vi "PECT - Scan_time gate.vi"() -> ()   [LabVIEW 2012]
uses:
  <vilib>/DAQmx/write.llb/DAQmx Write (Analog 1D Wfm NChan NSamp).vi
  <vilib>/DAQmx/read.llb/DAQmx Read (Analog 1D DBL 1Chan NSamp).vi
  <vilib>/DAQmx/read.llb/DAQmx Read (Analog Wfm 1Chan NSamp).vi
  <vilib>/Instr/_visa.llb/VISA Configure Serial Port (Instr).vi
  <vilib>/DAQmx/create/channels.llb/DAQmx Create Channel (AI-Voltage-Basic).vi
  <vilib>/DAQmx/configure/timing.llb/DAQmx Timing (Sample Clock).vi
  <vilib>/DAQmx/configure/task.llb/DAQmx Configure Logging (TDMS).vi
  <vilib>/DAQmx/configure/trigger.llb/DAQmx Start Trigger (Digital Edge).vi
  <vilib>/DAQmx/create/channels.llb/DAQmx Create Channel (AO-Voltage-Basic).vi
  <vilib>/DAQmx/miscellaneous.llb/DAQmx Fill In Error Info.vi
  Global_data.vi
  <vilib>/express/express analysis/Spectral/Block/exnSpectralBlock spectral measurements PSD poly.vi
  <vilib>/express/express analysis/Spectral/Block/exnSpectralBlock spectral measurements PSD WFM.vi
  <vilib>/express/express analysis/Spectral/XNode/ExpressSpectralMeasurementsBlockNode.xnode
  <resource>/objmgr/daqmx.rc
  <vilib>/measure/NI_MABase.lvlib
  <vilib>/Platform/NI_3dgraph.lvlib
panel:
  in  "Gate 2":dbl=2.0
  in  "Gate 1":dbl=4.0
  in  "Backward scan":bool
  in  "X-length count":dbl=20.0
  out "No.data":i32
  in  "Save Scan mode":bool caption="Save Process"
  in  "Plot style":i32(ring)=5 items=["cwLine"=1, "cwPoint"=2, "cwLinePoint"=3, "cwHiddenLine"=4, "cwSurface"=5, "cwSurfaceLine"=6, "cwSurfaceNormal"=7, "cwContourLine"=8, "cwSurfaceContour"=9]
  in  "Stop 4":bool
  in  "Forward scan":bool
  in  "ViewMode":i32(ring) items=["cwViewXYPlane", "cwViewXZPlane", "cwViewYZPlane", "cwViewUserDefined"]
  in  "Stop Scan 2":bool
  in  "Emergency Stop":bool
  in  "Stop 3":bool
  in  "Home Y":bool
  in  "Home X":bool
  in  "Back":bool
  in  "Front":bool
  in  "Left":bool
  in  "Right":bool
  in  "Stop Scan":bool
  in  "Move Distance (mm)":dbl=10.0
  in  "Scan":bool
  in  "Pulser Trigger Source":tag="/Dev1/PFI1" caption="소스"
  in  "Open":bool
  in  "Tab Control 2":T1(tab)
  out "Hall sensors signal":waveform(dbl)[](graph)=[{"t0"=timestamp(3525645621.636764 s since 1904-01-01), "dt"=1.9999999999999944e-06, "Y"=array[2100 elements], "attributes"=variant("NI_ChannelName"=variant(string "Dev1/ai0"), "NI_UnitDescription"=variant(string "Volts"))}, {"t0"=timestamp(3525645621.636764 s since 1904-01-01), "dt"=1.9999999999999944e-06, "Y"=array[2100 elements], "attributes"=variant("NI_ChannelName"=variant(string "Dev1/ai0"), "NI_UnitDescription"=variant(string "Volts"))}]
  out "Feature Extraction":dbl(graph)=0.021153968958947764
  out "Waveform Graph 2":waveform(dbl)[](graph)=[{"t0"=timestamp(0 s since 1904-01-01), "dt"=1.25e-06, "Y"=array[8000 elements]}]
  out "Power spectral density":cluster{"f0":dbl, "df":dbl, "magnitude":dbl[]}[](graph)=[{"f0"=0.0, "df"=238.09523809523876, "magnitude"=[-25.4340272409559, -28.495970805276507, -69.09064054555873, -79.11355871279994, -75.69366097931027, -84.18131507822396, -80.50168881348966, -82.72314293089615, -87.19630499623688, -82.83568021481967, -89.95290866002237, -85.90392585035596, -87.41269111550386, -91.40893948681482, -86.69370819914215, -93.36336146616782, -89.019380476413, -89.73232030153878, -94.58261196624535, -89.16287927388944, -94.965890302584, -91.86846413178648, -91.95327957161693, -97.62687167891286, -91.59993648735762, -97.30685711015555, -93.8350762480425, -93.27921214218685, -99.59438563802183, -93.1824258709588, -98.3113125531512, -95.45425138584356, -94.39327135467576, -100.65352961491782, -94.55889081970952, -99.40788907105079, -97.93617495318924, -96.19517579047603, -103.97036797797732, -96.40295202889732, -99.7036956909043, -99.48760137175819, -97.46192979187015, -106.29271483151813, -97.51447379981207, -99.86179280251669, -100.43811038443037, -97.59011642740829, -105.58363666166275, -99.01126121197593, -101.01575323613292, -101.90167607549864, -98.61952569586691, -106.73670466995647, -99.29976101634999, -101.54959604687718, -105.17330050767885, -100.09392305285375, -109.78264848704497, -100.98914236173123, -101.81665207962125, -105.42358374403365, -99.82880728595141, -107.07330885402075, -101.07712607444097, -101.03780825357597, -107.32811151840846, -101.221643458408, -105.63776326231454, -101.8420593566944, -101.80081629073969, -107.47915505307212, -101.12986632760553, -106.84901404755908, -102.73715610491038, -101.51552854007832, -107.28771371003282, -101.3928633472346, -107.44515355816633, -104.89304864643535, -103.1455098860718, -110.19910428997925, -102.73063833081197, -107.57101838377707, -104.90574568581201, -103.72599931018533, -109.97178587260123, -103.24611921258705, -108.36098023558972, -106.6408311450923, -104.73569536588386, -116.21683530762306, -105.02627439976544, -107.15856030450797, -109.81191038702062, -105.53476822084077, -119.10077766590356, -105.31867536160968, -106.9718410299748, -108.34458911268797, -104.70307996109247, -114.76704583683203, -106.29948298493936, -108.55077108437321, -112.16618350190343, -105.98453547558171, -114.68576835450673, -107.50968901677987, -107.89174277914348, -111.59875709602721, -106.69368240333122, -114.93273233954758, -105.23904516482949, -106.00272331017348, -110.36103151258544, -104.93177986717492, -110.8835476773746, -106.69346348818806, -106.66103973993782, -119.11729839814336, -108.06338160849775, -114.5879267769655, -108.59816838472844, -107.53189260743514, -114.07390818184973, -106.70996756049796, -113.27381274118753, -109.50270539577696, -107.37282420343303, -113.4779718725949, -106.04267666963091, -111.30294425571472, -112.46717993668915, -109.13164915488709, -116.65287200885172, -107.03002573045511, -110.21479040603631, -112.476075561056, -106.97710947409149, -119.42145279296255, -108.3200486628316, -110.46641858585929, -117.16650627564961, -109.73297826697552, -120.31689830731365, -107.19513745371916, -110.66663569403087, -113.30365980039964, -110.01971553524372, -123.68660617105166, -110.8171755739396, -111.11382172813546, -117.76239209582961, -109.49899370205401, -115.22252846498625, -111.1932077339224, -112.38235939086871, -118.22207022901702, -110.6546796895719, -116.97450780644367, -110.82401674194465, -111.96705198878843, -118.28092956599232, -110.5621503678909, -121.25720613496851, -111.98371482341479, -113.27928013246557, -111.96833712758355, -108.56859286664552, -120.32790468431601, -110.82699792221703, -110.79062667340345, -122.65756767769517, -110.48843456045427, -116.8782055296399, -115.43719816168479, -114.47619780315773, -121.42183196132746, -111.60631415727042, -120.68077308056417, -109.35478690141552, -109.03210709352732, -120.6260555904793, -109.47936424950136, -113.33719701518146, -112.88325992990137, -110.99901978536154, -123.19636626521421, -109.09861317900774, -113.33125158106256, -115.35673297389727, -112.77249677632989, -124.61163141716472, -114.68140920359865, -121.89642913325117, -115.47413298424323, -112.82196063671608, -127.87542521315149, -111.54178118788309, -113.6448752704395, -120.76569423868874, -112.98651214877823, -123.18868565400437, -115.41399838634062, -115.46853076016815, -116.40989072804102, -110.69611347288615, -132.23164080331392, -114.76376391429793, -121.7246597336247, -117.46893009589195, -114.01899156779395, -125.22079066032327, -114.59524199183258, -114.50034890537415, -122.9532092227648, -113.72727798159212, -125.65163915514907, -113.4793801211504, -110.4090756414644, -125.63592649005872, -114.22938378193007, -116.74947251106808, -121.60535557984142, -116.79385283402802, -122.44667696630361, -113.43873413563811, -123.28159708694415, -113.92892974938164, -114.01193823589753, -121.62751955742443, -118.76839573694522, -125.52998605097204, -115.19609643487229, -117.49409595176479, -117.08423885198002, -119.48314867245172, -125.01675515413412, -117.92668164142911, -115.55962389856793, -125.63488616674975, -119.11862859365166, -114.78860770332909, -117.18339781294443, -111.18063004722558, -118.31775966044624, -111.6867367949252, -114.57226159377, -119.36541212960576, -113.90245139442648, -132.46343443313128, -120.1282759002165, -121.05279009698619, -118.9115822659523, -121.23280439248342, -116.31914159559688, -127.38829313950257, -117.34673005740623, -115.95249861902771, -114.9301657394146, -123.22361802797445, -110.83274939062106, -116.16624248562111, -116.76753364192771, -113.94454545069023, -122.95736945775944, -118.66755800656253, -129.1462641201204, -116.6351050110328, -117.22529407303742, -123.80212197360244, -115.89792176423389, -114.25823938606595, -125.60467961977515, -114.59958849364433, -121.70071005514421, -118.25968972451209, -114.69929400946009, -123.88209034116528, -115.03869272537257, -117.52034211782204, -115.27990843516797, -117.85366603932033, -125.16865559622727, -118.21960424638507, -119.69008755413566, -117.24640963460672, -114.32867295013791, -119.1576982419508, -122.85495988425586, -116.3373010103401, -114.53730203699834, -115.67017599990201, -127.144321037601, -115.73849102686786, -117.7626163106355, -119.7346592991025, -117.41317517684553, -125.0417974461613, -114.5488949833583, -116.59812516173781, -119.91064563147799, -115.27933218667663, -122.09990513751134, -120.95678574143693, -123.25641714743752, -112.5173710452192, -113.53735878806998, -129.23914933506734, -116.27157269711533, -148.4020512032711, -118.84888216023774, -123.82550527215588, -116.87770979616658, -111.32191810025745, -124.32675905891588, -114.37182733794062, -121.10713785851372, -122.59698730059695, -116.38346694563282, -121.69144349152856, -119.00883142493832, -110.81886738196273, -120.7909830607913, -115.01780448665316, -114.52055121633796, -132.6824191654361, -116.330695115645, -126.4664151018508, -118.32717907779282, -118.7288071595281, -120.42749846140066, -112.53185615773879, -124.26026008984286, -114.24089252048742, -120.00368190003405, -114.71738500842926, -112.92262025927133, -129.21127897188563, -113.5947811765517, -117.80802009651353, -117.0133790103226, -112.19210322760304, -118.17549968071762, -119.3256187825503, -118.84981507334446, -121.39118969751144, -114.64543555194373, -119.84814933224528, -114.09123407848944, -116.22899352170892, -116.41650104077173, -113.70057202673476, -124.52773908304957, -114.87372641784933, -116.11651108221098, -121.68680962246994, -115.78306007961302, -122.22621008657796, -118.81157995182392, -113.9402115821658, -132.636729517989, -114.49554876936634, -119.50980190398928, -123.27410972236837, -118.52851881066383, -122.25212982572599, -117.13947036230024, -120.85005588797962, -118.41526503460501, -117.61788553858068, -126.3872056783977, -114.98198608543298, -119.7789938911847, -120.84873579392627, -114.38831474301695, -153.35954756825245, -113.19505610638078, -114.17454820985151, -127.41069917723112, -114.92677241657191, -125.49053973810628, -113.36382196587914, -119.96785250843519, -122.47388530423243, -116.38671253508838, -120.0905790211523, -119.83326265062107, -117.88168146696918, -122.3132169880757, -115.87324909105399, -125.92003267803432, -113.96860176867415, -114.49156118371398, -127.52634390035722, -115.05967156528004, -126.82020221981517, -117.93643187259194, -116.51163213641807, -119.47551219110167, -119.55225172256931, -116.9512257852571, -122.23153124485954, -120.8368476753637, -121.48473913072222, -115.83122660909913, -135.74260014140523, -116.58358375805423, -118.15236945484727, -119.06674062398864, -115.7844834762477, -125.06111738611818, -114.7801535050972, -115.2696605691888, -123.98656374010793, -119.29025555731172, -118.29146803784099, -119.55696172158135, -118.06884171238352, -127.81587648134607, -120.41730580797976, -123.49626136731604, -112.2147141798107, -116.22555232584983, -132.79419178871254, -119.66964883124663, -117.20946469243259, -118.20939292735417, -115.6951914646649, -129.64892855822356, -114.27056999288617, -120.31005512957381, -117.41846777372632, -115.50158386260813, -124.69777160737624, -115.2892897247205, -123.61522771666871, -113.75248734362687, -113.22999749252833, -129.3490509395313, -116.88137735661701, -116.94110280242681, -119.50244079984806, -119.30521139999144, -128.17199984115797, -118.06736594940236, -116.05331575995922, -121.29670750650897, -116.1140297602044, -125.090619084802, -121.41807296062154, -120.01332757902264, -120.54914530643151, -116.49738633175463, -122.32551291835904, -118.3190808346865, -118.92638453656723, -122.48819531011718, -117.01021725424317, -120.98896352560598, -117.23831688685218, -121.27915259197124, -121.20017251921661, -117.6155648860373, -120.91300272912063, -117.94438460863424, -115.94437430101533, -123.35904829443987, -117.74011174503076, -121.54935745388448, -120.82564553545025, -121.98951430455743, -120.24858103448778, -116.44403527138395, -112.79571494351876, -112.42801913096545, -110.1697573019791, -115.34500457736401, -119.81921052956707, -129.82600951154313, -115.5862301263047, -112.59292882433087, -120.79009137478283, -131.32849293387295, -113.61194478398238, -123.48568856527031, -119.17507777781304, -123.09261867490484, -116.97755217417308, -123.94453461434183, -116.58080525616379, -119.64289646280756, -122.90202645580743, -126.66219093058154, -121.95048829056148, -115.72578023509817, -116.70117814464484, -121.91050280869723, -118.25299095698178, -116.45905559047064, -132.57794493731578, -121.65327820443292, -120.9816664775787, -117.17270262269045, -120.27433984830965, -125.89418976028173, -119.09563505847817, -126.9693215534833, -113.17465524665704, -118.98702092883116, -119.83822568580342, -120.45832738089722, -120.67735960513633, -127.38676010839353, -127.65777338183055, -118.37446329057411, -115.61355494839711, -119.94568688114103, -116.06619937633681, -126.348857777089, -118.92850079147068, -119.5416617639739, -132.47075644221843, -118.08809356028496, -123.16186463092723, -121.51579486791232, -122.88983670053283, -129.5195538417256, -120.4730389608841, -132.16486858341602, -122.34690358436781, -120.71922104337597, -114.29260860841114, -117.67902631803368, -124.7040155514909, -123.51274592117205, -120.02297921674332, -136.54655493811157, -120.45629227407751, -119.06410204276258, -127.91681714792554, -122.82090055753153, -125.16838176650813, -121.79565386970478, -119.79607311590995, -126.54861375039647, -121.59135878113302, -132.8348640697562, -118.1305434733294, -120.46070148841905, -122.69571910896963, -117.6534954653865, -124.15742546824006, -120.73646926947502, -124.82696993800742, -124.513836786494, -123.15395713389651, -124.62395468806395, -117.21365768658171, -119.32635871968456, -121.48532284413152, -119.38242892643675, -126.25575652510352, -123.27133124029851, -117.58533922728374, -118.17710108929799, -114.99496360200965, -117.77133194647278, -111.34898201101595, -111.50817058307922, -119.0703124690998, -127.70676079885351, -121.8704969141074, -125.93154214283446, -118.65628450081473, -122.47918878348962, -117.9651589546518, -126.13560583004508, -122.42294805637847, -133.924453763793, -117.2082573038767, -117.6525335446734, -122.92077297426977, -122.04624645756786, -116.43289028226238, -117.93180959338378, -129.02356734231915, -117.95493621286326, -120.7555929766252, -120.76782849311112, -123.06287498470708, -117.83798593857965, -123.43423215434719, -120.15190119516652, -120.48240443128407, -143.29738987393452, -123.46572247444769, -120.89055325172792, -125.66715973809033, -118.26887578998644, -117.01836200028421, -121.33021830755509, -119.68846363313813, -122.60689066103069, -116.26858138914181, -119.59360791972998, -122.94866175463353, -114.174409515556, -118.00516930888391, -121.56978543579633, -135.87799017759036, -117.50816594504829, -122.82539428457626, -123.82103443155845, -124.77975840345442, -121.13340798086698, -120.93607435603558, -133.15787160745222, -120.70545628137863, -125.02155972441679, -122.04666465472178, -118.01234649746348, -127.88767491042842, -119.02096620167217, -120.16031065152875, -122.25406107859625, -121.72733059051095, -120.61357375519918, -118.63962847172827, -134.3857741605498, -116.3600853185034, -117.26695700691671, -119.9176982185873, -113.45576465218444, -126.69779573632724, -114.39554522802246, -116.8457146515868, -116.34219889483086, -119.30011291548334, -120.01163291843496, -114.29497178248809, -127.65687642749229, -119.58556923753022, -129.8593054181261, -122.2353645100479, -120.79536520223796, -119.83284028355028, -117.7991246185715, -128.390292904734, -119.78079925213122, -125.478913448993, -113.89747777944768, -112.66620124153357, -124.3475049842711, -120.85847303094337, -132.91807981902295, -119.523494985723, -116.65149909866443, -119.73287290436721, -127.63237851524192, -127.23413304048789, -120.87585453904362, -121.08540368080186, -134.91071939669257, -117.75375801669338, -117.2683014590723, -120.9739099492833, -118.23809733632451, -120.94065804928206, -123.88077510875804, -118.13812819300607, -122.60294123365466, -126.97075898006995, -120.18754789731035, -124.71238663441227, -120.55456557278582, -130.94599087480253, -111.18288669417035, -112.27708791831247, -126.0512034600378, -117.41881712783596, -128.20553880273903, -117.29482600885808, -118.2045526390752, -127.81966672699878, -117.03716165902529, -115.46711739757512, -117.15363929234843, -121.87599671671335, -121.19736800869221, -126.5301786755875, -131.20754947382918, -124.40138004810741, -129.0562496906515, -121.06816554587536, -121.01023627802867, -138.6137911215848, -120.12495002524031, -121.38510517514229, -122.79804220535513, -116.97501378195477, -118.82011581137473, -114.0229185604644, -119.54287501990726, -114.64474566771625, -117.76935669872461, -123.81082574158907, -118.51678358865587, -128.9664755188374, -123.45357998434133, -122.74888841574231, -120.74640581234044, -126.956344345126, -119.95682140104577, -118.8873101779055, -124.41062359284174, -128.97304498664363, -123.86287113204068, -127.30257087528216, -120.61364220528216, -114.45119129304715, -119.68384044686806, -131.29639185291157, -122.31250766293485, -119.57420865241102, -124.74014026002448, -124.87593035709094, -118.4566565612952, -123.76236085976001, -120.84780538841838, -117.68987599773281, -135.06195695255914, -122.56143585795171, -129.04610316842883, -118.32313199570537, -117.77093802786419, -124.46572845786741, -129.1123298336903, -120.88470269965448, -116.69988985752187, -116.84054667499878, -133.76883696987278, -122.32434984927302, -124.98940594457933, -122.56515592789917, -118.31562562243366, -133.97049179545627, -122.33220627999802, -131.16753675316977, -124.69828063969263, -116.37621154460467, -126.1833423168025, -129.62937634161355, -118.46241371150788, -117.52851478852457, -125.32425037236442, -119.0327364293772, -124.2861355894013, -123.24573502278234, -125.52155812053758, -113.75743410709823, -114.79513162658353, -128.58142362588052, -122.48277095196701, -118.94747544412269, -123.86988127835491, -124.78140456983323, -121.53998481875398, -116.01432822539552, -119.20174681160661, -122.75167725800814, -120.58657749420254, -118.51141061842183, -119.24457006171983, -131.43641234223372, -116.00759139055087, -121.24442216102587, -123.29371279953725, -117.608355420454, -116.33684374617326, -118.06291688281922, -121.88761866022774, -121.54820313120047, -119.5051369873635, -126.56611158390913, -118.84012713615805, -121.09285296522563, -124.67955377692547, -147.31451139022337, -116.80660421066897, -114.8367853755961, -120.41026468628925, -123.65666101895222, -119.64837119787269, -116.77480172559095, -116.54263359173909, -124.75286620868079, -117.33721912698883, -116.51795620907136, -118.50086748176733, -128.10381328920522, -122.78098994574157, -120.24716756092855, -119.52743204722819, -115.00407387659232, -108.2853711552629, -108.61086943894702, -119.6228894146785, -124.11132022420912, -125.6202218409766, -123.1749360787656, -118.1971196161698, -123.95075368058998, -121.72140109898365, -123.27106899042522, -123.73035629887062, -121.24369679109273, -121.07381526465288, -113.13965659723667, -118.330755475899, -118.40249076804484, -111.59630598649044, -116.1569506845575, -125.67326089915758, -125.85723567111906, -119.24293277595024, -117.87067617433537, -120.70936924059559, -131.8090588468898, -132.98711569625004, -123.63274249467587, -122.75476917502559, -126.12873814250243, -120.53144270605179, -129.07030822919336, -122.7889410422919, -124.35405971166259, -119.63968579420454, -139.0154441054289, -129.47962001806934, -121.86548015410847, -128.6818469257012, -121.40195873232601, -138.64231053781285, -124.22025721762265, -124.06073958736941, -126.71929802352521, -131.7498459276443, -120.68144109742178, -122.6325588818875, -126.80796617875095, -124.92487955227033, -136.94498040498806, -124.26704334219014, -123.21376211221711, -140.25352033075964, -129.53222319772195, -122.58541579060463, -122.1996729592375, -125.66642108013673, -125.66310429236694, -120.09682773706965, -125.27326633941439, -121.55721878725502, -121.22507119941083, -121.53716878624485, -136.20685498111987, -128.15260146013156, -120.03473972471616, -124.60755958763912, -124.73082500077143, -123.93425949983688, -131.04483249265184, -121.7957035014449, -127.09321441816094, -133.6144579272493, -124.69014595896968, -130.4902091211609, -121.18031440773905, -128.00033943961677, -125.88991118115149, -118.865310745079, -123.69668867733147, -117.98756965862728, -114.40013091842827, -118.28685032521078, -122.23464196869948, -124.8440422629961, -129.66281606870848, -119.440534215621, -124.54391783563877, -124.93447967158188, -121.7258558761523, -122.28817885403082, -127.06889620458577, -128.92172974939206, -120.62932166634072, -126.06847321900452, -123.31471168429935, -121.80350826545656, -129.2574604322076, -125.67225933193998, -125.7801671825605, -129.53804733161627, -119.56756644124712, -128.82490314699373, -124.7689736295626, -120.50019729114693, -124.50603158563972, -122.8120627011088, -125.60528875555717, -123.8817354922713, -124.05570537836674, -120.94568834491936, -118.06056028605255, -124.24390361274648, -125.5716703018188, -127.71949519914061, -130.7001652968252, -126.27701412017494, -133.76810134709916, -128.4738939614179, -120.302550881701, -118.91298143662928, -124.9077318110765, -127.16253699189492, -118.11405934812818, -117.52028071290711, -140.95620572748925, -123.61977932545628, -131.0334379970501, -125.88948384968432, -127.81552331993379, -121.92316280719056, -119.05911238768732, -126.83773251459189, -123.52627415002164, -120.8779561023192, -123.66683567603742, -131.64300993967345, -123.62895847772963, -116.89792951363142, -120.1068259250195, -117.92484706459337, -115.58208487778379, -120.76803581628594, -123.95408562090736, -122.79456549632754, -134.5305398779298, -123.57040300991032, -128.40634159414552, -123.70102187824159, -118.24970739397313, -119.66483900349026, -127.78024313111393, -120.3547204111785, -125.49305364308705, -119.49505591004302, -120.50920386196539, -119.03509516851003, -114.24667300009652, -121.60538636584391, -119.95304417598024, -122.24585853682832, -128.63653016912684, -116.04810628805795, -121.94159862131235, -122.59928204398939, -121.4532410501923, -128.6511474663462, -130.83715595958148, -121.71998300574741, -116.91426629511156, -113.587592058512, -115.59736707638731, -124.65300822631244, -133.32538684258748, -124.02289142873636, -121.54278890993639, -119.02596809402394, -108.90572887117857, -112.14974069608851, -129.21149299565423, -118.82148342951197, -116.65510894288538, -118.39609618084175, -116.53502642884725, -122.47549439965209, -122.23125657046063, -123.68081343116663, -120.67915071600007, -123.6899360128769, -118.56721985209728, -118.36641581191942, -126.96724630704657, -119.36877661672403, -123.07698921198843, -117.80772421906035, -122.82545076270567, -118.82755071380888, -117.21030132539394, -129.760567864525, -118.0816708063509, -125.80573274113647, -121.18434666182338, -121.80987210832065, -130.99259828357094, -125.47223579895922, -123.86818606677002, -118.7118158196511, -119.27778317338742, -127.27333258839096, -119.90672352079164, -140.78772370844268, -118.08251080057329, -119.86636232122572, -118.69482489738232, -119.19106512767372, -123.70988914879189, -121.92566832147995, -123.41378261726373, -120.1715186070818, -117.9079629421116, -117.41960207545632, -123.72833996166874, -127.24377206607298, -124.99098647980887, -129.48803701799955, -129.92351350561592, -120.79284154834647, -119.29601975194524, -136.17244775530037, -126.73975437546255, -128.84068276143336, -125.66374985701982, -136.69026010435715, -125.44409235146617, -119.28138070315057, -118.65017329869724, -118.02521532826772, -122.23736063759657, -121.27846943548622, -116.69850478126861, -119.7711336696722, -123.70776561180185, -118.43344549561263, -123.92390877157247, -117.19637143066551, -117.64112988205311, -127.78399195238529]}, ...(2 in all)]
  in  "3D Surface":refnum<k7>(container)
  out "Feature Extraction 2":dbl(graph)=0.021153968958947764
  out "Record path":path=path "D:/NDTENG/Foerster/ROTOMAT/Software/Roto_1.csv" caption="selected path"
  in  "Tab Control":T2(tab)
  out "No. X":i32
  out "No. Y":i32
  in  "X-length":dbl=20.0
  in  "Step X":dbl=0.2
  in  "COM Port":refnum<visa-resource-name>="COM1"
  in  "Baud Rate":u32=9600
  in  "Data bits":u16=8 min=5 max=8 step=1
  in  "stop bits":u16(ring)=10 items=["1.0"=10, "1.5"=15, "2.0"=20]
  in  "Parity":u16(ring) items=["None", "Odd", "Even", "Mark", "Space"]
  in  "1 Min":dbl=0.4
  in  "2 Max":dbl=6.0
  in  "1  Max":dbl=6.0
  in  "2 Min":dbl=0.4
  in  "Y-length":dbl=20.0
  in  "Step Y":dbl=0.2
  in  "1 Rate":dbl=0.2
  in  "2 Rate":dbl=0.4
  in  "Travel per Pulse (mm)":dbl=0.002
  in  "Cur. Pos X":dbl=-33.28 format="%#.4f"
  in  "Cur. Pos Y":dbl=30.0 format="%#.4f"
  in  "Save Speed":bool
  out "Move X":bool
  out "Sample per Channel AI":dbl
  out "Sample per Channel AO":dbl
  in  "Pulser Cycles":i32=10
  in  "Logging Mode":i32(ring)=10231 items=["Off"=10231, "Log and Read"=15842]
  out "Actual Sample Rate":dbl=500000.0 format="%0.2f"
  in  "Physical Channel":tag="Dev1/ai0"
  in  "Min Voltage":dbl=-10.0
  in  "Max Voltage":dbl=10.0
  in  "Terminal Configuration":i32(ring)=10083 items=["default"=-1, "RSE"=10083, "NRSE"=10078, "Differential"=10106, "Pseudodifferential"=12529]
  in  "Sample Clock Source 2":tag="OnboardClock"
  in  "Sample Rate":dbl=500000.0
  in  "TDMS File Path":path
  out "Actual Sample Rate 2":dbl=800000.0 format="%0.2f"
  in  "Physical Channel(s)":tag="Dev1/ao1"
  in  "Min Voltage 2":dbl=-10.0
  in  "Max Voltage 2":dbl=10.0
  in  "Sample Clock Source":tag="OnboardClock"
  in  "Sample Rate 2":dbl=800000.0
  in  "Offset":bool
  in  "2 Plots":bool
  in  "Edge":i32(ring)=10280 items=["Rising"=10280, "Falling"=10171]
  in  "Digital Trigger Source":tag="/Dev1/PFI0"
  in  "Duty cycle %":dbl=50.0 format="%#.2f"
  in  "Output Array":T3(array[cluster])=[{"Waveform Type"=2, "Amplitude"=10.0, "Frequency"=300.0}] {"Frequency" format="%0.2p"; "Amplitude" format="%0.2p"; "Waveform Type" items=["Sine Wave", "Triangle Wave", "Square Wave", "Sawtooth Wave"]}
  # "Pulse Shape"
  # "Trigger Settings"
  # "Data Processing"
  # "Time gate = T/xx"
  # "Pulse"
  # "Hall Sensors Signal"
  # "Feature Extraction"
  # "Power Spectal Density"
  # "COM  Setting"
  # "Speed  Setting"
  # "Scan  Setting"
  # "Pulse  Channel"
  # "Pulse  Timming"
  # "Sensor  Channel"
  # "DAQ Timming"
  # "Logging Settings"
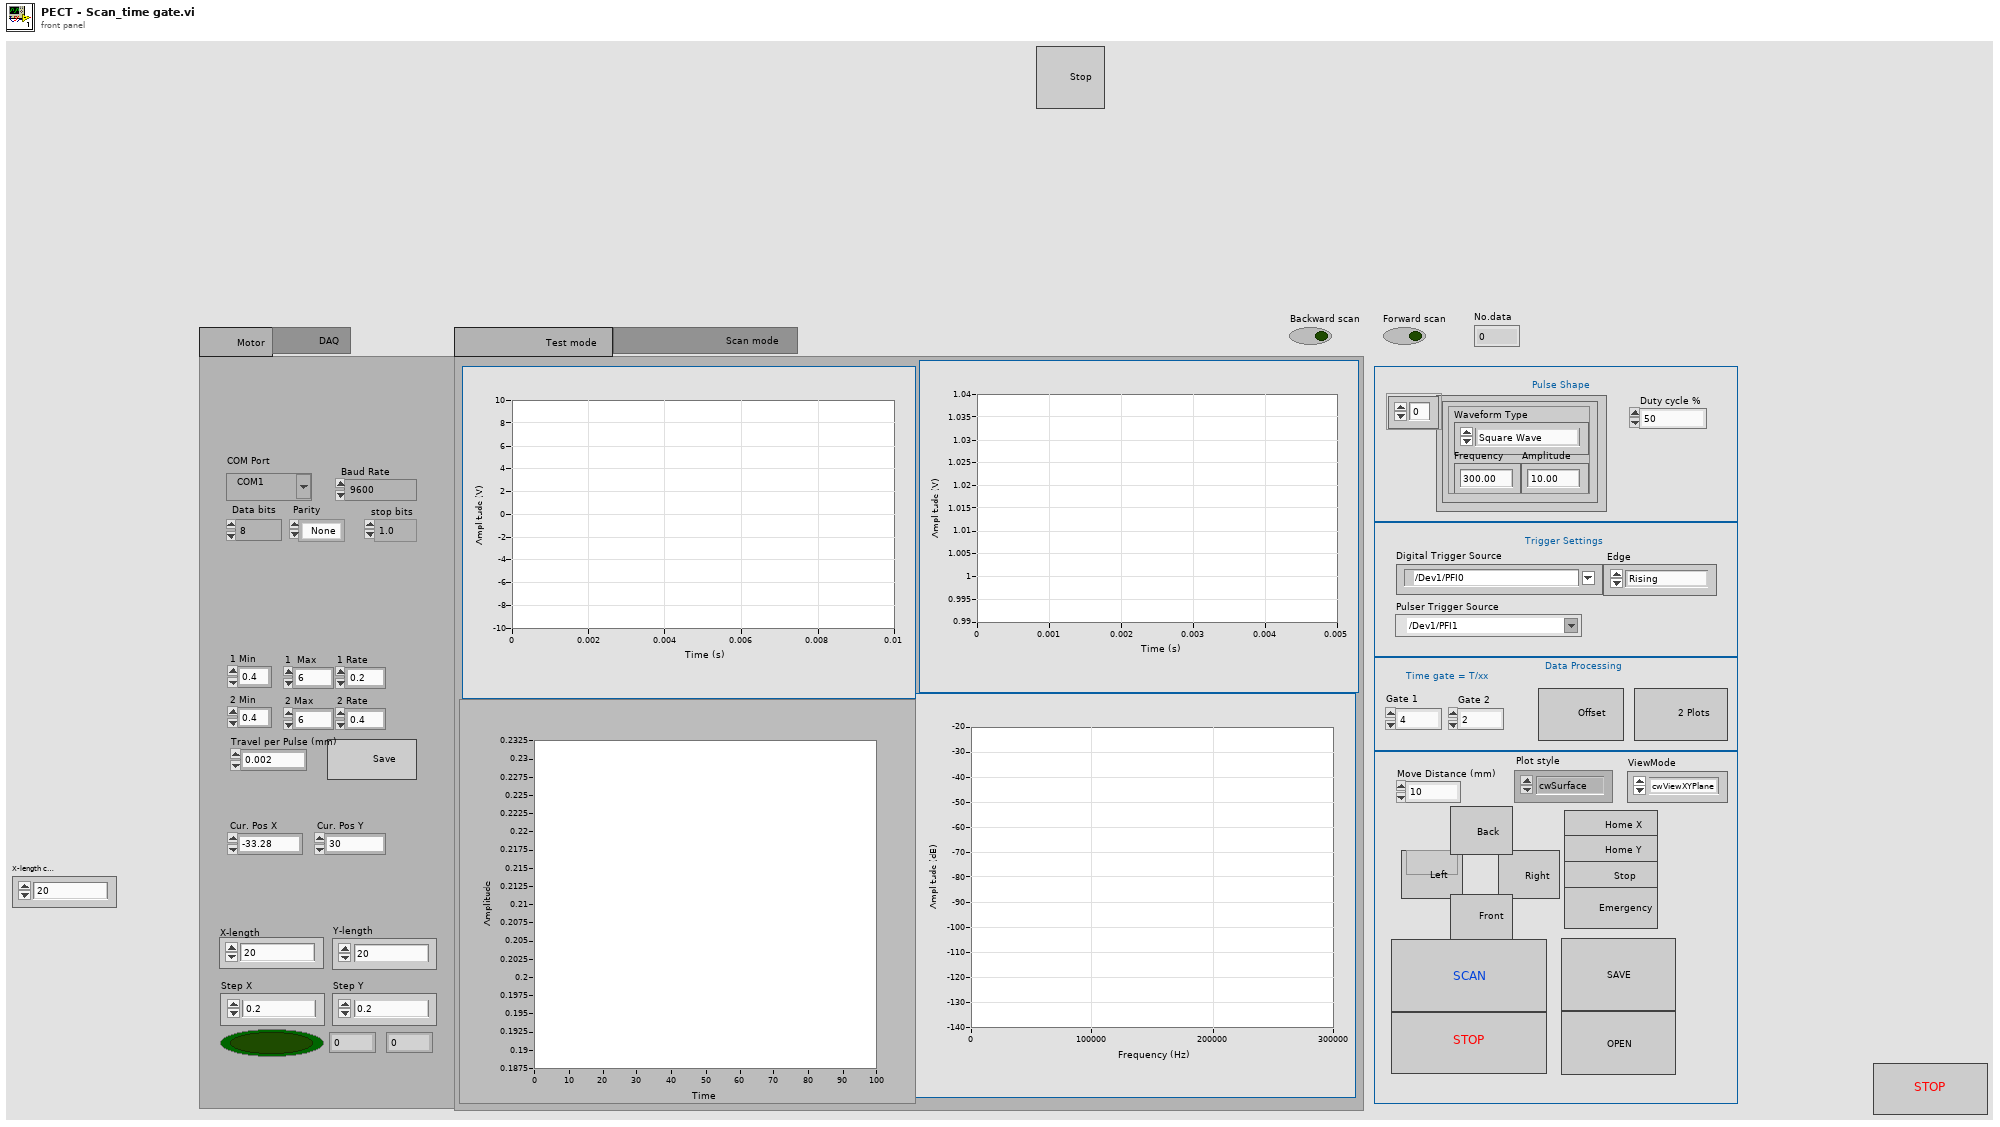
[diagram p1: front panel]
types:
  T1 = enum32{"                    Test mode                   ", "                          Scan mode                      "}
  T2 = enum32{"        Motor      ", "          DAQ        "}
  T3 = cluster{"Waveform Type":u16, "Amplitude":dbl, "Frequency":dbl}[]
  T4 = enum16{"open", "open or create", "create or replace", "create", "open (read-only)"}
  T5 = cluster{"Waveform Type":u16, "Amplitude":dbl, "Frequency":dbl}
  T6 = cluster{"averaging mode":u16, "weighting mode":u16, "number of averages":u32}
  T7 = cluster{"dB On (F)":bool, "unwrap phase (F)":bool, "convert to degree (F)":bool}
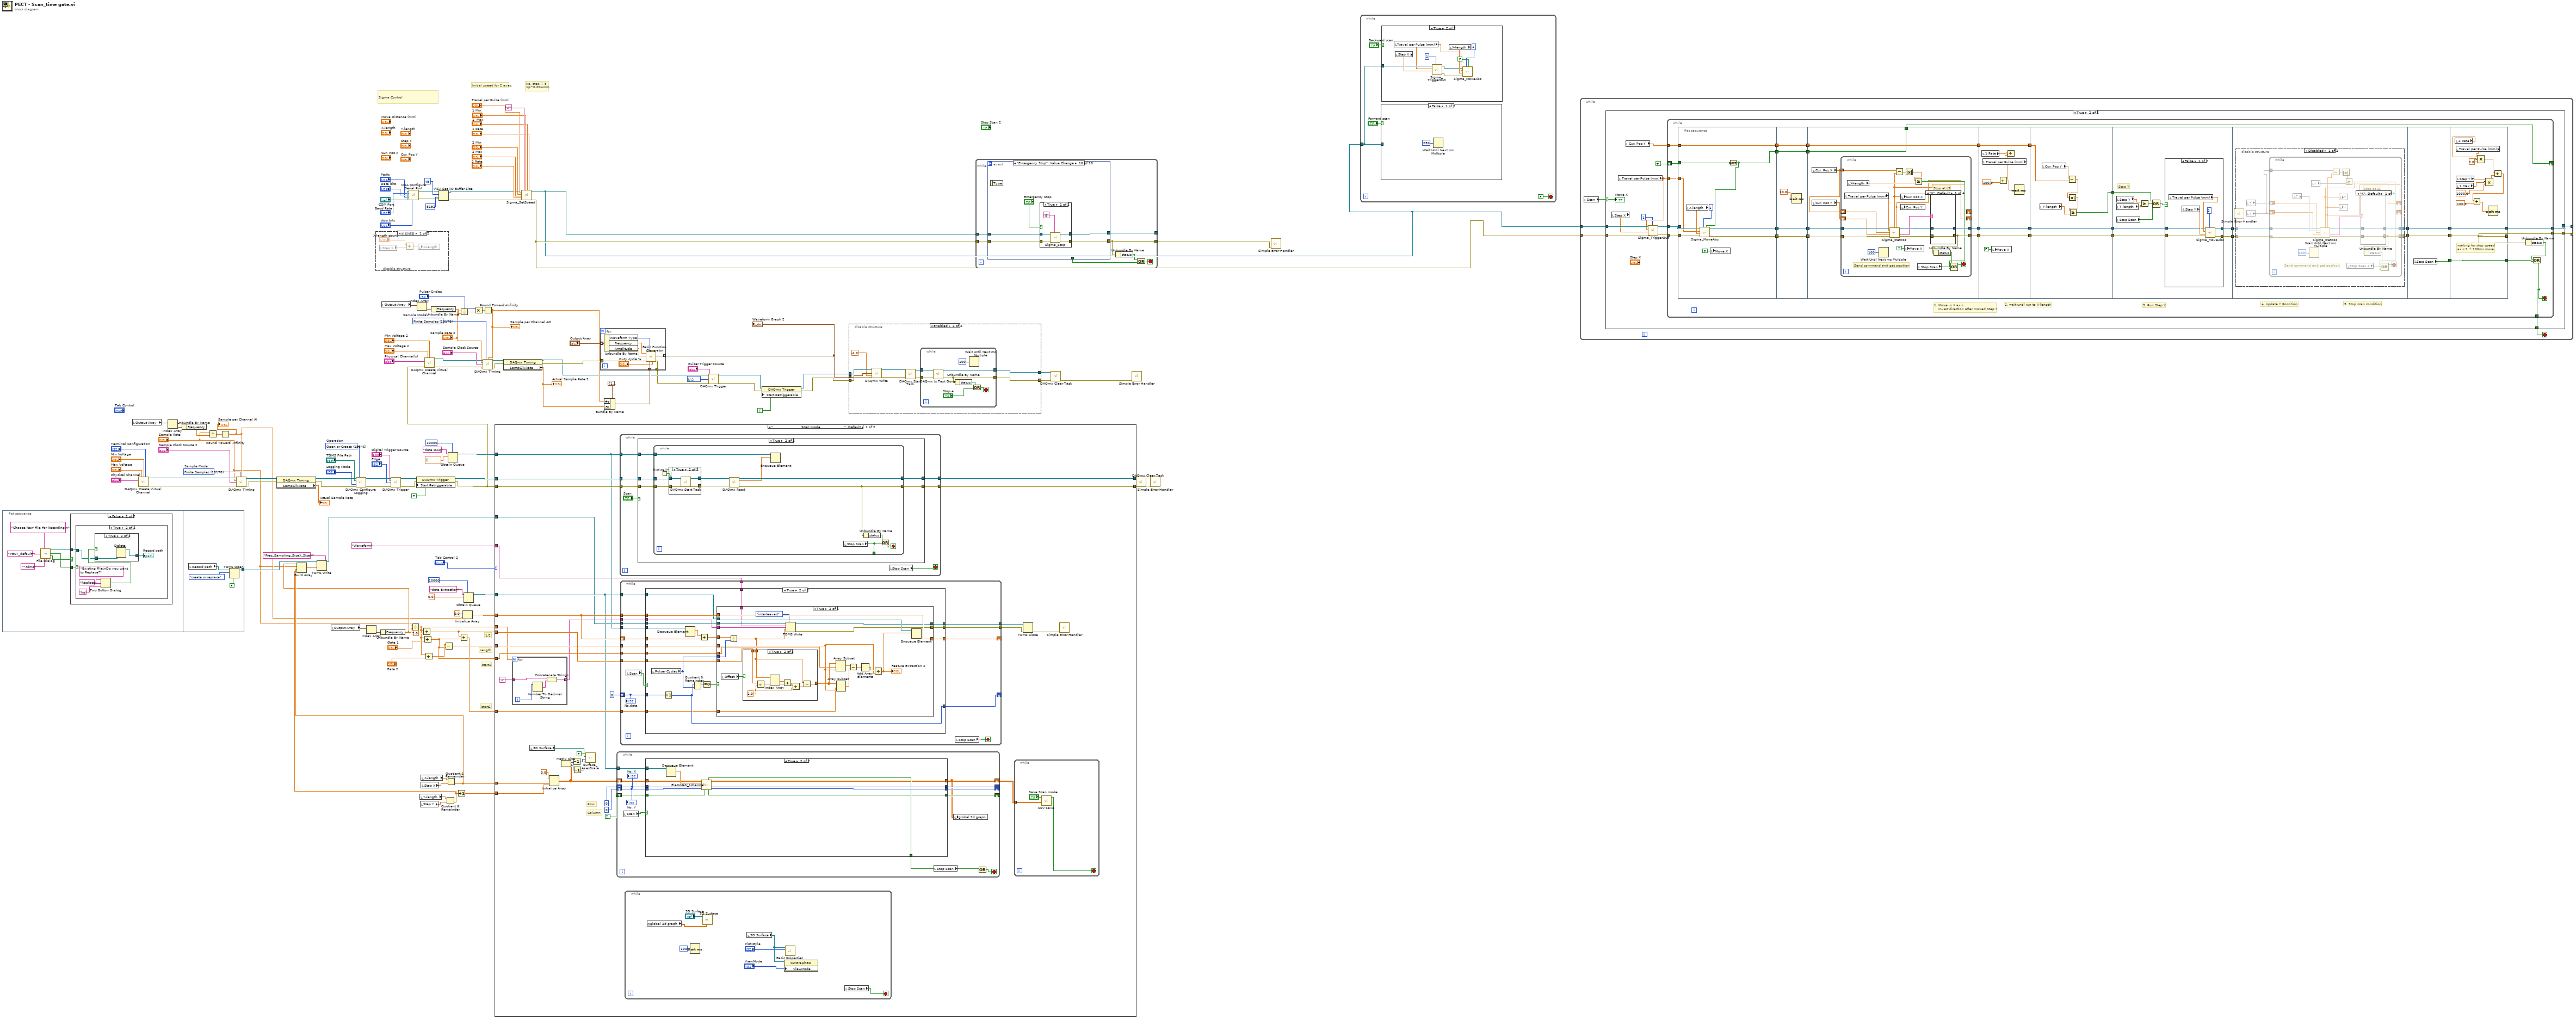
[diagram p0: block diagram]
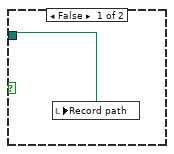
[diagram p2: hidden frame]
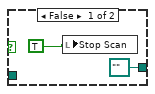
[diagram p3: hidden frame]
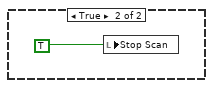
[diagram p4: hidden frame]
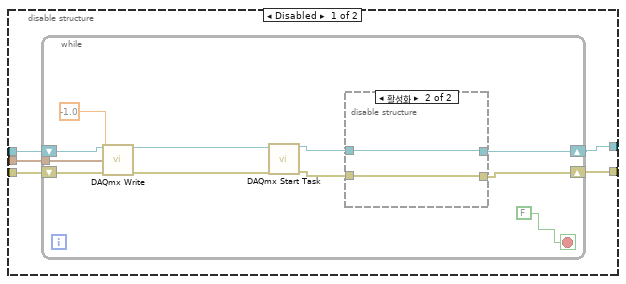
[diagram p6: hidden frame]
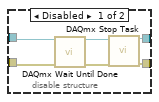
[diagram p7: hidden frame]
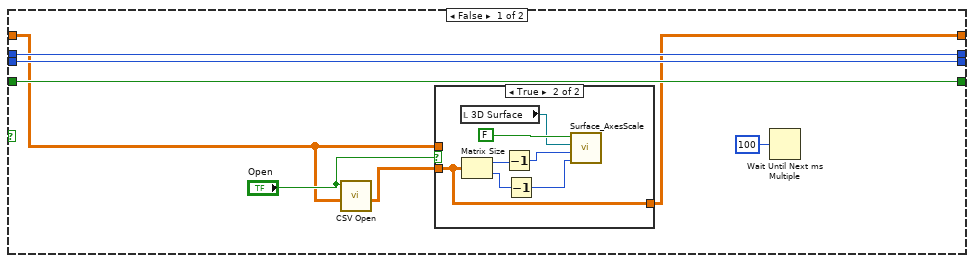
[diagram p8: hidden frame]
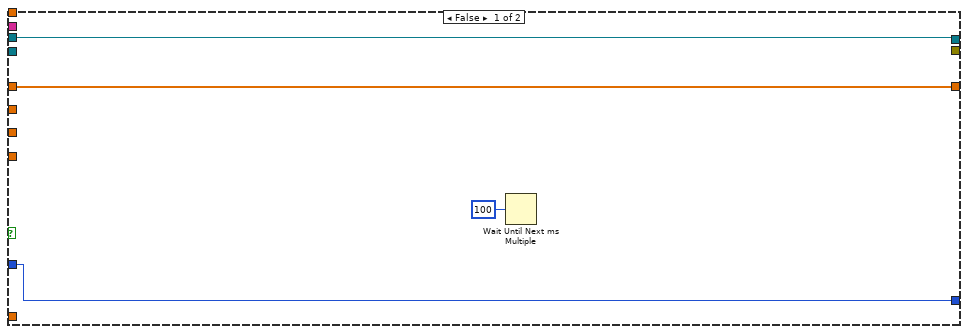
[diagram p12: hidden frame]
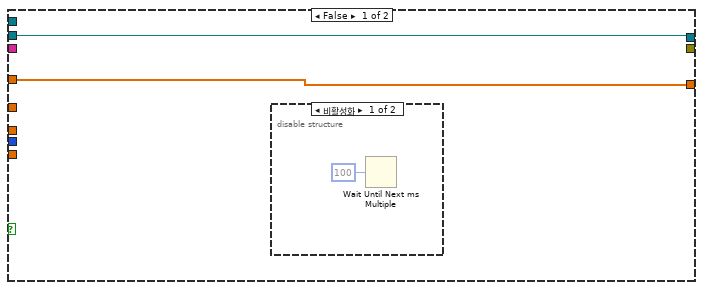
[diagram p13: hidden frame]
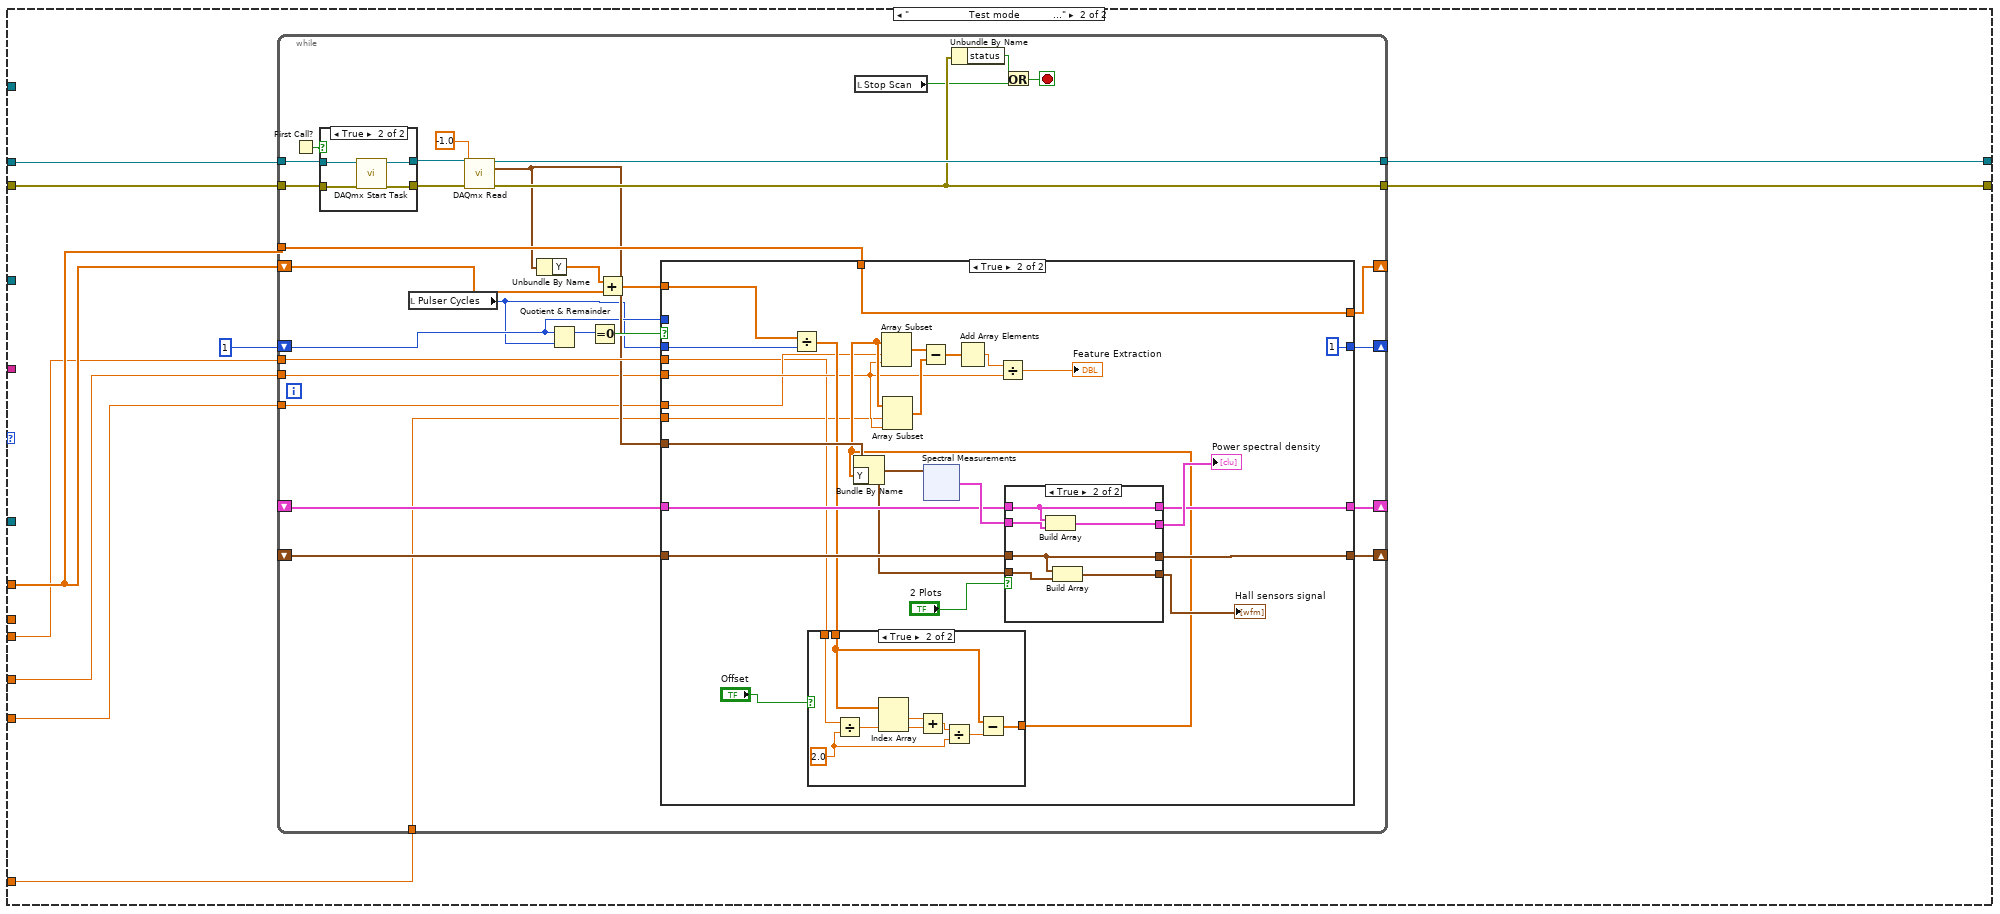
[diagram p16: hidden frame]
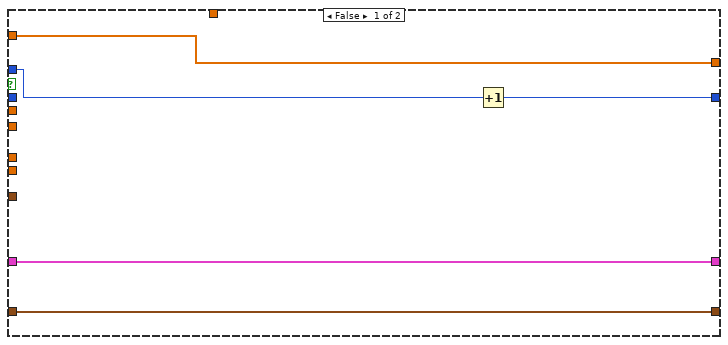
[diagram p18: hidden frame]
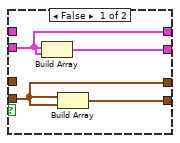
[diagram p20: hidden frame]
diagram:
  w43 = 10280 items=["상승"=10280, "하강"=10171] ("edge")
  w58 = 10178 items=["Finite Samples"=10178, "Continuous Samples"=10123, "Hardware Timed Single Point"=12522]  # Sample Mode
  w83 = 10178 items=["Finite Samples"=10178, "Continuous Samples"=10123, "Hardware Timed Single Point"=12522]  # Sample Mode
  w98 = 15846 items=["Open"=10437, "Open or Create"=15846, "Create or Replace"=15847, "Create"=15848]  # Operation
  # "1/2"
  # "start1"
  # "start2"
  # "Length"
  # "No. step = 5\n1p~0.004mm"
  # "Initial speed for 2 axes"
  # "Sigma Control"
  n1 = flat-sequence {
    tunnel: [w148] -> w10
    frame #0 {
      n2 = call "File Dialog"("prompt"="Choose New File For Recording\n" ("button label"), "default name"="PECT_default", "pattern (all files)"="*.tdms") -> ("selected path"=w132:path, "exists"=w127:bool, "cancelled"=w128:bool)  [unwired: 9 in, 1 out]
      n3 = case shown="False" w128 {
        tunnel: w132 -> [w133 _]
        tunnel: w127 -> [w134 _]
        frame False {
          n4 = case shown="True" w134 {
            tunnel: w133 -> [w135 w136]
            frame False {
              n5 = local write "Record path"(w135) -> ()
            }
            frame True {
              n6 = Two Button Dialog(message="Existing File\nDo you want to Replace?", 1:"No" ("F button name (\"Cancel\")"), 2:"Replace" ("T button name (\"OK\")")) -> (T button?=w137:bool)
              n7 = case shown="True" w137 {
                tunnel: w136 -> [_ w145]
                tunnel: [path "" ("deleted path") w144] -> w138
                frame False {
                  n8 = local write "Stop Scan"(TRUE ("Exit")) -> ()
                }
                frame True {
                  n9 = Delete(path (use dialog)=w145) -> (deleted path=w144:path)  [unwired: 4 in, 2 out]
                }
              }
              "Record path" <- w138
            }
          }
        }
        frame True {
          n10 = local write "Stop Scan"(TRUE ("Exit")) -> ()
        }
      }
    }
    frame #1 {
      n11 = local read "Record path"() -> (w147:path)
      n12 = TDMS Open(6:FALSE ("disable buffering (T)"), 10:T4."create or replace" ("operation"), 11:w147) -> (3:w148:refnum<k34>)  [unwired: 3 in, 1 out]
    }
  }
  n13 = local read "Output Array"() -> (w27:T3)
  n14 = call-poly <vilib>:"DAQmx Create Virtual Channel.vi"("maximum value"="Max Voltage", "minimum value"="Min Voltage", "input terminal configuration"="Terminal Configuration", "physical channels"="Physical Channel") -> ("task out"=w101:refnum<k21>, "error out"=w102:errorcluster)  [unwired: 10 in]
  n15 = Index Array(array=w27) -> (element=w25:T5)  [unwired: 1 in]
  n16 = Unbundle By Name(w25) -> ("Frequency"=w26:dbl)
  n17 = Divide(x="Sample Rate", y=w26) -> (x/y=w22:dbl)
  n18 = Round Toward -Infinity(1:w22) -> (0:w3:dbl)
  "Sample per Channel AI" <- w3
  n19 = call-poly <vilib>:"DAQmx Timing.vi"("task/channels in"=w101, "sample mode"=w83, "samples per channel"=w3, "rate"="Sample Rate", "source"="Sample Clock Source 2", "error in"=w102) -> ("task out"=w104:refnum<k21>, "error out"=w103:errorcluster)  [unwired: 8 in]
  n20 = property class="DAQmx Timing"(reference=w104, error in=w103) -> (reference out=w100:refnum<k21>, error out=w99:errorcluster, "SampClk.Rate"=→"Actual Sample Rate":dbl)
  n21 = local read "Output Array"() -> (w78:T3)
  n22 = call-poly <vilib>:"DAQmx Configure Logging.vi"("task/channels in"=w100, "operation"=w98, "file path"="TDMS File Path", "logging mode"="Logging Mode", "error in"=w99) -> ("task out"=w97:refnum<k21>, "error out"=w96:errorcluster)  [unwired: 9 in]
  n23 = Index Array(array=w78) -> (element=w77:T5)  [unwired: 1 in]
  n24 = disable-structure shown="비활성화" {
    frame Disabled {
      n25 = local read "Step X"() -> (w153:dbl)
      n26 = Add(x="X-length count", y=w153) -> (x+y=w152:dbl)
      n27 = local write "X-length"(w152) -> ()
    }
    frame Enabled {
    }
  }
  n28 = Unbundle By Name(w77) -> ("Frequency"=w4:dbl)
  n29 = local read "Output Array"() -> (w31:T3)
  n30 = call-poly <vilib>:"DAQmx Trigger.vi"("task/channels in"=w97, "source"="Digital Trigger Source", "edge"="Edge", "error in"=w96) -> ("task out"=w80:refnum<k21>, "error out"=w79:errorcluster)  [unwired: 10 in]
  n31 = call-poly "VISA Configure Serial Port"("VISA resource name"="COM Port", "baud rate (9600)"="Baud Rate", "data bits (8)"="Data bits", "parity (0:none)"="Parity", "stop bits (10: 1 bit)"="stop bits") -> ("VISA resource name out"=w113:refnum<visa-resource-name>, "error out"=w107:errorcluster)  [unwired: 9 in]
  n32 = Divide(x="Sample Rate", y=w4) -> (x/y=w1:dbl)
  n33 = property class="DAQmx Trigger"(reference=w80, error in=w79, "Start.Retriggerable"=TRUE) -> (reference out=w21:refnum<k21>, error out=w20:errorcluster)
  n34 = Index Array(array=w31) -> (element=w32:T5)  [unwired: 1 in]
  n35 = local read "Y-length"() -> (w64:dbl)
  n36 = local read "Step Y"() -> (w65:dbl)
  n37 = local read "X-length"() -> (w67:dbl)
  n38 = local read "Step X"() -> (w66:dbl)
  n39 = Divide(x=w1, y=2.0) -> (x/y=w17:dbl)
  n40 = Divide(x=w1, y="Gate 1") -> (x/y=w13:dbl)
  n41 = Divide(x=w1, y="Gate 2") -> (x/y=w14:dbl)
  n42 = call-poly <vilib>:"DAQmx Create Virtual Channel.vi"("maximum value"="Max Voltage 2", "minimum value"="Min Voltage 2", "physical channels"="Physical Channel(s)", "error in"=w20) -> ("task out"=w42:refnum<k21>, "error out"=w41:errorcluster)  [unwired: 10 in]
  n43 = Unbundle By Name(w32) -> ("Frequency"=w33:dbl)
  n44 = VISA Set I/O Buffer Size(VISA resource name=w113, mask (16)=48, size (4096)=u32 8192, error in (no error)=w107) -> (VISA resource name out=w117:refnum<visa-resource-name>, error out=w116:errorcluster)
  n45 = Subtract(x=w14, y=w13) -> (x-y=w15:dbl)
  n46 = Quotient & Remainder(x=w64, y=w65) -> (floor(x/y)=w6:dbl)  [unwired: 1 out]
  n47 = Quotient & Remainder(x=w67, y=w66) -> (floor(x/y)=w8:dbl)  [unwired: 1 out]
  n48 = Build Array(w4, "Sample Rate", w8, w6) -> (w11:dbl[])
  n49 = TDMS Write(0:w10, 5:"Freq_Sampling_SizeX_SizeY" ("group name in (Untitled)"), 9:w11) -> (4:w9:refnum<k34>)  [unwired: 3 in, 3 out]
  n50 = Obtain Queue(max queue size (-1, unlimited)=10000, name (unnamed)="data DAQ", element data type=dbl[] [] ("data")) -> (queue out=w72:refnum<queue>)  [unwired: 2 in, 2 out]
  n51 = Increment(x=w6) -> (x+1=w7:dbl)
  n52 = Add(x=w17, y=w13) -> (x+y=w16:dbl)
  n53 = Divide(x="Sample Rate 2", y=w33) -> (x/y=w29:dbl)
  n54 = Initialize Array(0.0 ("element"), w3) -> (w73:dbl[])
  n55 = Obtain Queue(max queue size (-1, unlimited)=10000, name (unnamed)="data Extraction", element data type=0.0) -> (queue out=w70:refnum<queue>)  [unwired: 2 in, 2 out]
  n56 = Multiply(x="Pulser Cycles", y=w29) -> (x*y=w24:dbl)
  n57 = Round Toward -Infinity(1:w24) -> (0:w23:dbl)
  "Sample per Channel AO" <- w23
  n58 = call-poly <vilib>:"DAQmx Timing.vi"("task/channels in"=w42, "sample mode"=w58, "samples per channel"=w23, "rate"="Sample Rate 2", "source"="Sample Clock Source", "error in"=w41) -> ("task out"=w60:refnum<k21>, "error out"=w59:errorcluster)  [unwired: 8 in]
  n59 = case shown="\"                          Scan mode                      \", Default" "Tab Control 2" {
    tunnel: w21 -> [w187 w361]
    tunnel: [w186 w360] -> w86
    tunnel: [w185 w359] -> w85
    tunnel: w73 -> [w182 w358]
    tunnel: w20 -> [w184 w357]
    tunnel: w17 -> [w183 w356]
    tunnel: w72 -> [w181 _]
    tunnel: w70 -> [w173 _]
    tunnel: w8 -> [w156 _]
    tunnel: w7 -> [w179 _]
    tunnel: w15 -> [w165 w354]
    tunnel: w13 -> [w164 w353]
    tunnel: w16 -> [w163 w352]
    tunnel: w9 -> [w162 _]
    tunnel: "Waveform" ("group name in (Untitled)") -> [w159 _]
    tunnel: w1 -> [w155 _]
    frame "                          Scan mode                      ", Default {
      # "Column"
      # "Row"
      n60 = for {
        N: w155 -> [_]
        tunnel: "X" -> [w189]
        tunnel: [w188] -> w154 mode=indexing
        i -> [w191]
        n61 = Number To Decimal String(number=w191) -> (decimal integer string=w190:string)  [unwired: 1 in]
        n62 = Concatenate Strings(w189, w190) -> (w188:string)
      }
      n63 = local read "3D Surface"() -> (w166:refnum<k7>)
      n64 = Initialize Array(0.0 ("element"), w156, w179) -> (w172:dbl[][])
      n65 = Matrix Size(0:w172) -> (1:w174:i32, 2:w175:i32)
      n66 = Decrement(x=w174) -> (x-1=w178:i32)
      n67 = Decrement(x=w175) -> (x-1=w177:i32)
      n68 = call "Surface_AxesScale.vi"("Y-axis Max"=w177, "X-axis max"=w178, "3D Surface"=w166, "Auto Scale"=FALSE) -> ()  [unwired: 8 in]
      n69 = while {
        shift-right: [w212] -> _
        shift-left: 0 -> [w214]
        shift-right: [w211] -> _
        shift-left: 0 -> [w213]
        tunnel: w173 -> [w210]
        shift-right: [w202] -> w167
        shift-left: w172 -> [w209]
        shift-right: [w203] -> _
        shift-left: TRUE ("Output Direction") -> [w204]
        stop <- w206 stop-if-true
        n70 = local read "Scan"() -> (w208:bool)
        n71 = case shown="True" w208 {
          tunnel: w214 -> [w222 w241]
          tunnel: w213 -> [w221 w240]
          tunnel: [w222 w239] -> w212
          tunnel: [w221 w238] -> w211
          tunnel: w210 -> [_ w237]
          tunnel: w209 -> [w216 w235]
          tunnel: [w215 w231] -> w202
          tunnel: [_ w234] -> w205
          tunnel: w204 -> [w220 w233]
          tunnel: [w220 w232] -> w203
          frame False {
            n72 = call "CSV Open.vi"("2D Array In"=w216, "Open"="Open") -> ("2D Array Out"=w219:dbl[][])  [unwired: 9 in]
            n73 = case shown="True" "Open" {
              tunnel: w219 -> [_ w225]
              tunnel: [w223 w225] -> w215
              tunnel: w216 -> [w223 _]
              frame False {
              }
              frame True {
                n74 = local read "3D Surface"() -> (w224:refnum<k7>)
                n75 = Matrix Size(0:w225) -> (1:w226:i32, 2:w227:i32)
                n76 = Decrement(x=w226) -> (x-1=w230:i32)
                n77 = Decrement(x=w227) -> (x-1=w229:i32)
                n78 = call "Surface_AxesScale.vi"("Y-axis Max"=w229, "X-axis max"=w230, "3D Surface"=w224, "Auto Scale"=FALSE) -> ()  [unwired: 8 in]
              }
            }
            n79 = Wait Until Next ms Multiple(millisecond multiple=u32 100 ("ms 배수")) -> ()  [unwired: 1 out]
          }
          frame True {
            n80 = Dequeue Element(queue=w237) -> (element=w236:dbl)  [unwired: 2 in, 3 out]
            n81 = call "EletoMatr_1channel.vi"("Input Array X"=w235, "Input data"=w236, "In Row"=w241, "In Column"=w240, "Input Direction"=w233) -> ("Completed"=w234:bool, "Out Array X"=w231:dbl[][], "Out Row"=w239:i32, "Output Direction"=w232:bool, "Out Column"=w238:i32)  [unwired: 6 in]
          }
        }
        n82 = local read "Stop Scan"() -> (w207:bool)
        n83 = global write "Global_data.vi" "global 2d graph"(w202) -> ()
        n84 = Compound Arithmetic op=OR(w205, w207) -> (w206:bool)
        "No. Y" <- w213
        "No. X" <- w214
      }
      n85 = while {
        tunnel: w187 -> [w248]
        tunnel: [w247] -> w186
        tunnel: [w246] -> w185
        tunnel: w184 -> [w245]
        tunnel: w181 -> [w244]
        stop <- w243 stop-if-true
        n86 = case shown="True" "Scan" {
          tunnel: w248 -> [w250 w255]
          tunnel: [w250 w254] -> w247
          tunnel: [w249 w253] -> w246
          tunnel: w245 -> [w249 w252]
          tunnel: w244 -> [_ w251]
          frame False {
          }
          frame True {
            n87 = while {
              tunnel: w255 -> [w261]
              tunnel: [w267] -> w254
              tunnel: [w266] -> w253
              tunnel: w252 -> [w260]
              tunnel: w251 -> [w265]
              tunnel: [w262] -> _
              stop <- w263 stop-if-true
              n88 = First Call?() -> (First Call?: T/F=w257:bool)
              n89 = case shown="True" w257 {
                tunnel: w261 -> [w268 w273]
                tunnel: w260 -> [w269 w272]
                tunnel: [w268 w271] -> w259
                tunnel: [w269 w270] -> w258
                frame False {
                }
                frame True {
                  n90 = call <vilib>:"DAQmx Start Task.vi"("task/channels in"=w273, "error in"=w272) -> ("task out"=w271:refnum<k21>, "error out"=w270:errorcluster)  [unwired: 12 in]
                }
              }
              n91 = call-poly <vilib>:"DAQmx Read.vi"("task/channels in"=w259, "error in"=w258) -> ("task out"=w267:refnum<k21>, "data"=w256:dbl[], "error out"=w266:errorcluster)  [unwired: 11 in]
              n92 = Enqueue Element(queue=w265, element=w256) -> ()  [unwired: 2 in, 3 out]
              n93 = local read "Stop Scan"() -> (w262:bool)
              n94 = Unbundle By Name(w266) -> ("status"=w264:bool)
              n95 = Or(x=w264, y=w262) -> (x .or. y?=w263:bool)
            }
          }
        }
        n96 = local read "Stop Scan"() -> (w243:bool)
      }
      n97 = while {
        shift-right: [w287] -> _
        shift-left: w182 -> [w291]
        tunnel: w182 -> [w290]
        tunnel: w183 -> [w289]
        tunnel: w181 -> [w288]
        tunnel: w173 -> [w286]
        shift-right: [w283] -> _
        shift-left: 0 -> [w284]
        tunnel: w165 -> [w281]
        tunnel: w164 -> [w280]
        tunnel: w163 -> [w279]
        tunnel: w162 -> [w278]
        tunnel: [w277] -> w161
        tunnel: [w276] -> w160
        tunnel: w159 -> [w275]
        tunnel: w154 -> [w274]
        stop <- w282 stop-if-true
        n98 = local read "Scan"() -> (w285:bool)
        n99 = case shown="True" w285 {
          tunnel: w291 -> [w295 w307]
          tunnel: w290 -> [_ w313]
          tunnel: w289 -> [_ w312]
          tunnel: w288 -> [_ w311]
          tunnel: [w295 w310] -> w287
          tunnel: w286 -> [_ w309]
          tunnel: w284 -> [w294 w305]
          tunnel: [w294 w304] -> w283
          tunnel: w281 -> [_ w303]
          tunnel: w280 -> [_ w302]
          tunnel: w279 -> [_ w301]
          tunnel: w278 -> [w292 w300]
          tunnel: [w292 w299] -> w277
          tunnel: [_ w298] -> w276
          tunnel: w275 -> [_ w297]
          tunnel: w274 -> [_ w296]
          frame False {
            n100 = Wait Until Next ms Multiple(millisecond multiple=u32 100 ("ms 배수")) -> ()  [unwired: 1 out]
          }
          frame True {
            n101 = local read "Pulser Cycles"() -> (w306:i32)
            n102 = Increment(x=w305) -> (x+1=w304:i32)
            n103 = Dequeue Element(queue=w311) -> (element=w308:dbl[])  [unwired: 2 in, 3 out]
            n104 = Quotient & Remainder(x=w304, y=w306) -> (x-y*floor(x/y)=w314:i32)  [unwired: 1 out]
            n105 = Add(x=w308, y=w307) -> (x+y=w316:dbl[])
            n106 = Equal To 0?(x=w314) -> (x = 0?=w315:bool)
            n107 = case shown="True" w315 {
              tunnel: w306 -> [_ w336]
              tunnel: w316 -> [w318 w326]
              tunnel: [w318 w341] -> w310
              tunnel: w313 -> [_ w341]
              tunnel: w312 -> [_ w330]
              tunnel: w309 -> [_ w334]
              tunnel: w303 -> [_ w331]
              tunnel: w302 -> [_ w328]
              tunnel: w301 -> [_ w329]
              tunnel: w300 -> [w317 w327]
              tunnel: [w317 w325] -> w299
              tunnel: [_ w324] -> w298
              tunnel: w297 -> [_ w323]
              tunnel: w296 -> [_ w320]
              frame False {
                n108 = disable-structure shown="비활성화" {
                  frame Disabled {
                    n109 = Wait Until Next ms Multiple(millisecond multiple=u32 100 ("ms 배수")) -> ()  [unwired: 1 out]
                  }
                  frame Enabled {
                  }
                }
              }
              frame True {
                n110 = local read "Offset"() -> (w333:bool)
                n111 = Divide(x=w326, y=w336) -> (x/y=w322:dbl[])
                n112 = case shown="True" w333 {
                  tunnel: w330 -> [_ w350]
                  tunnel: w322 -> [w342 w344]
                  tunnel: [w342 w343] -> w335
                  frame False {
                  }
                  frame True {
                    w346 = 2.0 ("y")
                    n113 = Divide(x=w350, y=w346) -> (x/y=w351:dbl)
                    n114 = Index Array(array=w344, index #2=w351) -> (element #1=w348:dbl, element #2=w349:dbl)  [unwired: 1 in]
                    n115 = Add(x=w348, y=w349) -> (x+y=w347:dbl)
                    n116 = Divide(x=w347, y=w346) -> (x/y=w345:dbl)
                    n117 = Subtract(x=w344, y=w345) -> (x-y=w343:dbl[])
                  }
                }
                n118 = TDMS Write(0:w327, 1:enum16{"decimated", "interleaved"}."interleaved" ("데이터 레이아웃(0:decimated)"), 5:w323, 7:w320, 9:w322) -> (4:w325:refnum<k34>, 15:w324:errorcluster)  [unwired: 1 in, 2 out]
                n119 = Array Subset(array=w335, index=w328, length=w331) -> (w339:dbl[])
                n120 = Array Subset(array=w335, index=w329, length=w331) -> (w338:dbl[])
                n121 = Subtract(x=w339, y=w338) -> (x-y=w337:dbl[])
                n122 = Add Array Elements(numeric array=w337) -> (sum=w340:dbl)
                n123 = Divide(x=w340, y=w331) -> (x/y=w332:dbl)
                "Feature Extraction 2" <- w332
                n124 = Enqueue Element(queue=w334, element=w332) -> ()  [unwired: 2 in, 3 out]
              }
            }
          }
        }
        n125 = local read "Stop Scan"() -> (w282:bool)
        "No.data" <- w284
      }
      n126 = while {
        stop <- w196 stop-if-true
        n127 = global read "Global_data.vi" "global 2d graph"() -> (w192:dbl[][])
        n128 = Wait (ms)(milliseconds to wait=u32 100) -> ()  [unwired: 1 out]
        n129 = call <vilib>:"3D Surface.vi"("z matrix"=w192, "3D graph"="3D Surface") -> ()  [unwired: 8 in, 2 out]
        n130 = local read "3D Surface"() -> (w198:refnum<k7>)
        n131 = property class="CWGraph3D"(reference=w198, "ViewMode"="ViewMode") -> ()  [unwired: 1 in, 2 out]
        n132 = call <vilib>:"Basic Properties.vi"("3D graph"=w198, "plot style"="Plot style") -> ()  [unwired: 12 in, 2 out]
        n133 = local read "Stop Scan"() -> (w196:bool)
      }
      n134 = while {
        tunnel: w167 -> [w200]
        stop <- w199 stop-if-true
        n135 = call "CSV Save.vi"("Array"=w200, "Save Button"="Save Scan mode") -> ("Save Status"=w199:bool)  [unwired: 9 in]
      }
      n136 = TDMS Close(8:w160, 11:w161) -> (0:w158:errorcluster)  [unwired: 1 out]
      n137 = call <vilib>:"Simple Error Handler.vi"("error in (no error)"=w158) -> ()  [unwired: 2 in, 7 out]
    }
    frame "                    Test mode                   " {
      n138 = while {
        tunnel: w361 -> [w368]
        tunnel: w357 -> [w367]
        tunnel: [w389] -> w359
        tunnel: [w390] -> w360
        shift-right: [w384] -> _
        shift-left: w358 -> [w385]
        tunnel: w358 -> [w383]
        shift-right: [w381] -> _
        shift-left: _ -> [w380]
        tunnel: w356 -> [w379]
        shift-right: [w378] -> _
        shift-left: _ -> [w377]
        shift-right: [w372] -> _
        shift-left: 1 ("Average") -> [w371]
        tunnel: w354 -> [w364]
        tunnel: w353 -> [w363]
        tunnel: w352 -> [w362]
        stop <- w391 stop-if-true
        n139 = First Call?() -> (First Call?: T/F=w369:bool)
        n140 = case shown="True" w369 {
          tunnel: w368 -> [w392 w397]
          tunnel: w367 -> [w393 w396]
          tunnel: [w392 w395] -> w366
          tunnel: [w393 w394] -> w365
          frame False {
          }
          frame True {
            n141 = call <vilib>:"DAQmx Start Task.vi"("task/channels in"=w397, "error in"=w396) -> ("task out"=w395:refnum<k21>, "error out"=w394:errorcluster)  [unwired: 12 in]
          }
        }
        n142 = local read "Pulser Cycles"() -> (w370:i32)
        n143 = call-poly <vilib>:"DAQmx Read.vi"("task/channels in"=w366, "timeout"=-1.0, "error in"=w365) -> ("task out"=w390:refnum<k21>, "data"=w373:waveform(dbl), "error out"=w389:errorcluster)  [unwired: 10 in]
        n144 = Unbundle By Name(w373) -> ("Y"=w376:dbl[])
        n145 = Quotient & Remainder(x=w371, y=w370) -> (x-y*floor(x/y)=w387:i32)  [unwired: 1 out]
        n146 = Equal To 0?(x=w387) -> (x = 0?=w386:bool)
        n147 = Add(x=w376, y=w385) -> (x+y=w382:dbl[])
        n148 = case shown="True" w386 {
          tunnel: w370 -> [_ w408]
          tunnel: w373 -> [_ w428]
          tunnel: w382 -> [w402 w427]
          tunnel: [w402 w426] -> w384
          tunnel: w383 -> [_ w426]
          tunnel: [w401 w422] -> w381
          tunnel: w380 -> [w401 w424]
          tunnel: w379 -> [_ w404]
          tunnel: [w400 w417] -> w378
          tunnel: w377 -> [w400 w419]
          tunnel: [w398 1 ("Average")] -> w372
          tunnel: w371 -> [w399 _]
          tunnel: w364 -> [_ w406]
          tunnel: w363 -> [_ w405]
          tunnel: w362 -> [_ w403]
          frame False {
            n149 = Increment(x=w399) -> (x+1=w398:i32)
          }
          frame True {
            n150 = Divide(x=w427, y=w408) -> (x/y=w411:dbl[])
            n151 = case shown="True" "Offset" {
              tunnel: w404 -> [_ w437]
              tunnel: w411 -> [w429 w431]
              tunnel: [w429 w430] -> w409
              frame False {
              }
              frame True {
                w433 = 2.0 ("y")
                n152 = Divide(x=w437, y=w433) -> (x/y=w438:dbl)
                n153 = Index Array(array=w431, index #2=w438) -> (element #1=w435:dbl, element #2=w436:dbl)  [unwired: 1 in]
                n154 = Add(x=w435, y=w436) -> (x+y=w434:dbl)
                n155 = Divide(x=w434, y=w433) -> (x/y=w432:dbl)
                n156 = Subtract(x=w431, y=w432) -> (x-y=w430:dbl[])
              }
            }
            n157 = Bundle By Name(cluster=w428, "Y"=w409) -> (w416:waveform(dbl))
            n158 = Array Subset(array=w409, index=w405, length=w406) -> (w415:dbl[])
            n159 = Array Subset(array=w409, index=w403, length=w406) -> (w414:dbl[])
            n160 = Subtract(x=w415, y=w414) -> (x-y=w413:dbl[])
            n161 = xnode "Spectral Measurements"("신호"=w416) -> ("PSD"=w420:cluster{"f0":dbl, "df":dbl, "magnitude":dbl[]})  [unwired: 1 in, 1 out]
            n162 = Add Array Elements(numeric array=w413) -> (sum=w421:dbl)
            n163 = Divide(x=w421, y=w406) -> (x/y=→"Feature Extraction":dbl)
            n164 = case shown="True" "2 Plots" {
              tunnel: [w442 w448] -> w425
              tunnel: w424 -> [_ w447]
              tunnel: [w441 w447] -> w422
              tunnel: w416 -> [w441 w443]
              tunnel: w420 -> [w439 w445]
              tunnel: [w440 w446] -> w418
              tunnel: w419 -> [_ w444]
              tunnel: [w439 w444] -> w417
              frame False {
                n165 = Build Array(w439, w439) -> (w440:cluster{"f0":dbl, "df":dbl, "magnitude":dbl[]}[])
                n166 = Build Array(w441, w441) -> (w442:waveform(dbl)[])
              }
              frame True {
                n167 = Build Array(w444, w445) -> (w446:cluster{"f0":dbl, "df":dbl, "magnitude":dbl[]}[])
                n168 = Build Array(w447, w443) -> (w448:waveform(dbl)[])
              }
            }
            "Power spectral density" <- w418
            "Hall sensors signal" <- w425
          }
        }
        n169 = local read "Stop Scan"() -> (w375:bool)
        n170 = Unbundle By Name(w389) -> ("status"=w388:bool)
        n171 = Or(x=w388, y=w375) -> (x .or. y?=w391:bool)
      }
    }
  }
  n172 = property class="DAQmx Timing"(reference=w60, error in=w59) -> (reference out=w46:refnum<k21>, error out=w52:errorcluster, "SampClk.Rate"=w50:dbl)
  "Actual Sample Rate 2" <- w50
  n173 = call "Sigma_SetSpeed.vi"("VISA resource name"=w117, "Travel per Pulse (0.004mm)"="Travel per Pulse (mm)", "Min (1mm) 2"="2 Min", "Max (2mm) 2"="2 Max", "Rate (1mm) 2"="2 Rate", "error in (no error)"=w116, "Axis (1)"="W", "Min (1mm)"="1 Min", "Max (2mm)"="1  Max", "Rate (1mm)"="1 Rate") -> ("VISA resource name out"=w105:refnum<visa-resource-name>, "error out"=w106:errorcluster)  [unwired: 8 in]
  n174 = Bundle By Name(cluster=cluster{"Fs":dbl, "#s":dbl} {"Fs"=1000.0, "#s"=1000.0} ("sampling info"), "#s"=w23, "Fs"=w50) -> (w49:cluster{"Fs":dbl, "#s":dbl})
  n175 = for {
    tunnel: w52 -> [w466]
    tunnel: w49 -> [w465]
    tunnel: [w464] -> w45
    tunnel: "Output Array" -> [w463] mode=indexing
    tunnel: [w460] -> w48 mode=indexing
    n176 = Unbundle By Name(w463) -> ("Waveform Type"=w462:u16, "Frequency"=w461:dbl, "Amplitude"=w458:dbl)
    n177 = call <vilib>:"Basic Function Generator.vi"("square wave duty cycle (%)"="Duty cycle %", "sampling info"=w465, "signal type"=w462, "error in (no error)"=w466, "amplitude"=w458, "frequency"=w461) -> ("error out"=w464:errorcluster, "signal out"=w460:waveform(dbl))  [unwired: 3 in, 1 out]
  }
  "Waveform Graph 2" <- w48
  n178 = call-poly <vilib>:"DAQmx Trigger.vi"("task/channels in"=w46, "source"="Pulser Trigger Source", "edge"=w43, "error in"=w45) -> ("task out"=w38:refnum<k21>, "error out"=w34:errorcluster)  [unwired: 10 in]
  n179 = property class="DAQmx Trigger"(reference=w38, error in=w34, "Start.Retriggerable"=TRUE) -> (reference out=w37:refnum<k21>, error out=w36:errorcluster)
  n180 = disable-structure shown="Enabled" {
    disable-tunnel: w48 -> [w471 w494]
    disable-tunnel: [w470 w493] -> w40
    disable-tunnel: [w469 w492] -> w39
    disable-tunnel: w37 -> [w468 w496]
    disable-tunnel: w36 -> [w467 w495]
    frame Disabled {
      n181 = while {
        tunnel: w471 -> [w482]
        shift-right: [w478] -> w470
        shift-left: w468 -> [w476]
        shift-right: [w477] -> w469
        shift-left: w467 -> [w475]
        stop <- FALSE stop-if-true
        n182 = call-poly <vilib>:"DAQmx Write.vi"("task/channels in"=w476, "data"=w482, "timeout"=-1.0, "error in"=w475) -> ("task out"=w481:refnum<k21>, "error out"=w480:errorcluster)  [unwired: 9 in, 1 out]
        n183 = call <vilib>:"DAQmx Start Task.vi"("task/channels in"=w481, "error in"=w480) -> ("task out"=w474:refnum<k21>, "error out"=w473:errorcluster)  [unwired: 12 in]
        n184 = disable-structure shown="활성화" {
          disable-tunnel: [w488 w490] -> w478
          disable-tunnel: [w487 w489] -> w477
          disable-tunnel: w474 -> [w486 w490]
          disable-tunnel: w473 -> [w485 w489]
          frame Disabled {
            n185 = call <vilib>:"DAQmx Wait Until Done.vi"("task/channels in"=w486, "error in"=w485) -> ("task out"=w484:refnum<k21>, "error out"=w483:errorcluster)  [unwired: 12 in]
            n186 = call <vilib>:"DAQmx Stop Task.vi"("task/channels in"=w484, "error in"=w483) -> ("task out"=w488:refnum<k21>, "error out"=w487:errorcluster)  [unwired: 12 in]
          }
          frame Enabled {
          }
        }
      }
    }
    frame Enabled {
      n187 = call-poly <vilib>:"DAQmx Write.vi"("task/channels in"=w496, "data"=w494, "timeout"=-1.0, "error in"=w495) -> ("task out"=w498:refnum<k21>, "error out"=w500:errorcluster)  [unwired: 9 in, 1 out]
      n188 = call <vilib>:"DAQmx Start Task.vi"("task/channels in"=w498, "error in"=w500) -> ("task out"=w497:refnum<k21>, "error out"=w499:errorcluster)  [unwired: 12 in]
      n189 = while {
        tunnel: w497 -> [w508]
        tunnel: w499 -> [w507]
        tunnel: [w505] -> w492
        tunnel: [w506] -> w493
        stop <- w501 stop-if-true
        n190 = call <vilib>:"DAQmx Is Task Done.vi"("task/channels in"=w508, "error in"=w507) -> ("task out"=w506:refnum<k21>, "error out"=w505:errorcluster)  [unwired: 11 in, 1 out]
        n191 = Unbundle By Name(w505) -> ("status"=w502:bool)
        n192 = Wait Until Next ms Multiple(millisecond multiple=u32 100) -> ()  [unwired: 1 out]
        n193 = Compound Arithmetic op=OR(w502, "Stop 4") -> (w501:bool)
      }
    }
  }
  n194 = while {
    tunnel: w105 -> [w515]
    tunnel: [w510] -> _
    tunnel: w106 -> [w514]
    tunnel: [w512] -> w126
    stop <- w511 stop-if-true
    n195 = event shown="[9] \"Emergency Stop\": Value Change" {
      selector: _ -> [_ _ _ _ _ _ _ _ _ _]
      dyn-events: _ -> [_ _ _ _ _ _ _ _ _ _]
      timeout: _ -> [_ _ _ _ _ _ _ _ _ _]
      tunnel: w515 -> [w517 w530 w533 w548 w563 w578 w595 w607 w617 w629]
      tunnel: w514 -> [w516 w527 w532 w547 w562 w577 w594 w606 w616 w628]
      tunnel: [w517 w529 w535 w550 w565 w580 w592 w605 w619 w631] -> w510
      tunnel: [w516 w528 w534 w549 w564 w579 w591 w604 w618 w630] -> w512
      tunnel: ["Stop Scan" _ _ _ _ _ _ _ _ _] -> w509
      event "Stop Scan": Value Change {
        n196 = event-data() -> ()  [unwired: 1 in, 2 out]
      }
      event "Save Speed": Value Change {
        n197 = event-data() -> ()  [unwired: 1 in, 5 out]
        n198 = local read "Travel per Pulse (mm)"() -> (w519:dbl)
        n199 = local read "1  Max"() -> (w524:dbl)
        n200 = local read "1 Rate"() -> (w523:dbl)
        n201 = local read "2 Rate"() -> (w520:dbl)
        n202 = local read "2 Max"() -> (w521:dbl)
        n203 = local read "1 Min"() -> (w525:dbl)
        n204 = local read "2 Min"() -> (w522:dbl)
        n205 = call "Sigma_SetSpeed.vi"("VISA resource name"=w530, "Travel per Pulse (0.004mm)"=w519, "Min (1mm) 2"=w522, "Max (2mm) 2"=w521, "Rate (1mm) 2"=w520, "error in (no error)"=w527, "Axis (1)"="W", "Min (1mm)"=w525, "Max (2mm)"=w524, "Rate (1mm)"=w523) -> ("VISA resource name out"=w529:refnum<visa-resource-name>, "error out"=w528:errorcluster)  [unwired: 8 in]
      }
      event "Right": Value Change {
        n206 = event-data() -> ()  [unwired: 1 in, 1 out]
        n207 = case shown="True" "Right" {
          tunnel: [w537 w543] -> w535
          tunnel: [w536 w542] -> w534
          tunnel: w533 -> [w537 w545]
          tunnel: w532 -> [w536 w544]
          frame False {
          }
          frame True {
            n208 = local read "Travel per Pulse (mm)"() -> (w539:dbl)
            n209 = local read "Move Distance (mm)"() -> (w538:dbl)
            n210 = call "Sigma_MoveAbs.vi"("Direction (+)"=FALSE, "Axis (1)"=1, "error in (no error)"=w544, "Travel (1mm)"=w538, "Travel per Pulse (0.004mm)"=w539, "VISA resource name"=w545) -> ("error out"=w542:errorcluster, "VISA resource name out"=w543:refnum<visa-resource-name>)  [unwired: 4 in]
          }
        }
      }
      event "Left": Value Change {
        n211 = event-data() -> ()  [unwired: 1 in, 1 out]
        n212 = case shown="True" "Left" {
          tunnel: [w552 w559] -> w550
          tunnel: [w551 w558] -> w549
          tunnel: w548 -> [w552 w560]
          tunnel: w547 -> [w551 w557]
          frame False {
          }
          frame True {
            n213 = local read "Travel per Pulse (mm)"() -> (w554:dbl)
            n214 = local read "Move Distance (mm)"() -> (w553:dbl)
            n215 = call "Sigma_MoveAbs.vi"("Direction (+)"=TRUE, "Axis (1)"=1, "error in (no error)"=w557, "Travel (1mm)"=w553, "Travel per Pulse (0.004mm)"=w554, "VISA resource name"=w560) -> ("error out"=w558:errorcluster, "VISA resource name out"=w559:refnum<visa-resource-name>)  [unwired: 4 in]
          }
        }
      }
      event "Front": Value Change {
        n216 = event-data() -> ()  [unwired: 1 in, 1 out]
        n217 = case shown="True" "Front" {
          tunnel: [w567 w573] -> w565
          tunnel: [w566 w572] -> w564
          tunnel: w563 -> [w567 w575]
          tunnel: w562 -> [w566 w574]
          frame False {
          }
          frame True {
            n218 = local read "Travel per Pulse (mm)"() -> (w569:dbl)
            n219 = local read "Move Distance (mm)"() -> (w568:dbl)
            n220 = call "Sigma_MoveAbs.vi"("Direction (+)"=FALSE, "Axis (1)"=2, "error in (no error)"=w574, "Travel (1mm)"=w568, "Travel per Pulse (0.004mm)"=w569, "VISA resource name"=w575) -> ("error out"=w572:errorcluster, "VISA resource name out"=w573:refnum<visa-resource-name>)  [unwired: 4 in]
          }
        }
      }
      event "Back": Value Change {
        n221 = event-data() -> ()  [unwired: 1 in, 1 out]
        n222 = case shown="True" "Back" {
          tunnel: [w582 w588] -> w580
          tunnel: [w581 w587] -> w579
          tunnel: w578 -> [w582 w590]
          tunnel: w577 -> [w581 w589]
          frame False {
          }
          frame True {
            n223 = local read "Travel per Pulse (mm)"() -> (w584:dbl)
            n224 = local read "Move Distance (mm)"() -> (w583:dbl)
            n225 = call "Sigma_MoveAbs.vi"("Direction (+)"=TRUE, "Axis (1)"=2, "error in (no error)"=w589, "Travel (1mm)"=w583, "Travel per Pulse (0.004mm)"=w584, "VISA resource name"=w590) -> ("error out"=w587:errorcluster, "VISA resource name out"=w588:refnum<visa-resource-name>)  [unwired: 4 in]
          }
        }
      }
      event "Home X": Value Change {
        n226 = event-data() -> ()  [unwired: 1 in, 1 out]
        n227 = case shown="True" "Home X" {
          tunnel: [w597 w600] -> w592
          tunnel: [w596 w599] -> w591
          tunnel: w595 -> [w597 w602]
          tunnel: w594 -> [w596 w601]
          frame False {
          }
          frame True {
            n228 = call "Sigma_Home.vi"("Axis (1)"="1", "error in (no error)"=w601, "VISA resource name"=w602) -> ("error out"=w599:errorcluster, "VISA resource name out"=w600:refnum<visa-resource-name>)  [unwired: 7 in]
          }
        }
      }
      event "Home Y": Value Change {
        n229 = event-data() -> ()  [unwired: 1 in, 1 out]
        n230 = case shown="True" "Home Y" {
          tunnel: [w609 w612] -> w605
          tunnel: [w608 w611] -> w604
          tunnel: w607 -> [w609 w614]
          tunnel: w606 -> [w608 w613]
          frame False {
          }
          frame True {
            n231 = call "Sigma_Home.vi"("Axis (1)"="2", "error in (no error)"=w613, "VISA resource name"=w614) -> ("error out"=w611:errorcluster, "VISA resource name out"=w612:refnum<visa-resource-name>)  [unwired: 7 in]
          }
        }
      }
      event "Stop 3": Value Change {
        n232 = event-data() -> ()  [unwired: 1 in, 1 out]
        n233 = case shown="True" "Stop 3" {
          tunnel: [w621 w622] -> w619
          tunnel: [w620 w623] -> w618
          tunnel: w617 -> [w621 w625]
          tunnel: w616 -> [w620 w624]
          frame False {
          }
          frame True {
            n234 = call "Sigma_Stop.vi"("Axis (1)"="W", "error in (no error)"=w624, "VISA resource name"=w625) -> ("error out"=w623:errorcluster, "VISA resource name out"=w622:refnum<visa-resource-name>)  [unwired: 7 in]
          }
        }
      }
      event "Emergency Stop": Value Change {
        n235 = event-data() -> ()  [unwired: 1 in, 1 out]
        n236 = case shown="True" "Emergency Stop" {
          tunnel: [w633 w636] -> w631
          tunnel: [w632 w635] -> w630
          tunnel: w629 -> [w633 w638]
          tunnel: w628 -> [w632 w637]
          frame False {
          }
          frame True {
            n237 = call "Sigma_Stop.vi"("Axis (1)"="E", "error in (no error)"=w637, "VISA resource name"=w638) -> ("error out"=w635:errorcluster, "VISA resource name out"=w636:refnum<visa-resource-name>)  [unwired: 7 in]
          }
        }
      }
    }
    n238 = Unbundle By Name(w512) -> ("status"=w513:bool)
    n239 = Compound Arithmetic op=OR(w513, w509) -> (w511:bool)
  }
  n240 = call <vilib>:"DAQmx Clear Task.vi"("task in"=w40, "error in"=w39) -> ("error out"=w57:errorcluster)  [unwired: 13 in]
  n241 = call <vilib>:"Simple Error Handler.vi"("error in (no error)"=w57) -> ()  [unwired: 4 in, 5 out]
  n242 = call <vilib>:"DAQmx Clear Task.vi"("task in"=w86, "error in"=w85) -> ("error out"=w95:errorcluster)  [unwired: 13 in]
  n243 = call <vilib>:"Simple Error Handler.vi"("error in (no error)"=w95) -> ()  [unwired: 4 in, 5 out]
  n244 = call <vilib>:"Simple Error Handler.vi"("error in (no error)"=w126) -> ()  [unwired: 4 in, 5 out]
  n245 = while {
    tunnel: w105 -> [w639]
    stop <- FALSE stop-if-true
    n246 = case shown="False" "Forward scan" {
      tunnel: w639 -> [_ w655]
      frame False {
        n247 = Wait Until Next ms Multiple(millisecond multiple=u32 250 ("ms 배수")) -> ()  [unwired: 1 out]
      }
      frame True {
        n248 = local read "Travel per Pulse (mm)"() -> (w654:dbl)
        n249 = local read "Step X"() -> (w660:dbl)
        n250 = call "Sigma_TriggerOut.vi"("Axis(1)"=1, "Trigger distance (mm)"=w660, "Travel per Pulse (mm)"=w654, "VISA resource name"=w655) -> ("error out"=w656:errorcluster, "VISA resource name out"=w657:refnum<visa-resource-name>)  [unwired: 6 in]
        n251 = local read "X-length"() -> (w658:dbl)
        n252 = call "Sigma_MoveAbs.vi"("Axis (1)"=1, "error in (no error)"=w656, "Travel (1mm)"=w658, "Travel per Pulse (0.004mm)"=w654, "VISA resource name"=w657) -> ()  [unwired: 5 in, 2 out]
      }
    }
    n253 = case shown="True" "Backward scan" {
      tunnel: w639 -> [_ w646]
      frame False {
        n254 = Wait Until Next ms Multiple(millisecond multiple=u32 250 ("ms 배수")) -> ()  [unwired: 1 out]
      }
      frame True {
        n255 = local read "Travel per Pulse (mm)"() -> (w645:dbl)
        n256 = local read "Step X"() -> (w651:dbl)
        n257 = call "Sigma_TriggerOut.vi"("Axis(1)"=1, "Trigger distance (mm)"=w651, "Travel per Pulse (mm)"=w645, "VISA resource name"=w646) -> ("error out"=w647:errorcluster, "VISA resource name out"=w648:refnum<visa-resource-name>)  [unwired: 6 in]
        n258 = local read "X-length"() -> (w649:dbl)
        n259 = call "Sigma_MoveAbs.vi"("Direction (+)"=FALSE, "Axis (1)"=1, "error in (no error)"=w647, "Travel (1mm)"=w649, "Travel per Pulse (0.004mm)"=w645, "VISA resource name"=w648) -> ()  [unwired: 4 in, 2 out]
      }
    }
  }
  n260 = while {
    tunnel: w105 -> [w667]
    tunnel: [w665] -> _
    tunnel: w106 -> [w666]
    tunnel: [w664] -> _
    stop <- w663 stop-if-true
    n261 = local read "Scan"() -> (w662:bool)
    n262 = case shown="True" w662 {
      selector: w662 -> [_ w713]
      tunnel: [w669 w715] -> w665
      tunnel: w667 -> [w671 w712]
      tunnel: w666 -> [w670 w709]
      tunnel: [w668 w714] -> w664
      tunnel: [FALSE w717] -> w663
      frame False {
        n263 = while {
          tunnel: w670 -> [w680]
          tunnel: [w675] -> w669
          tunnel: [w674] -> w668
          tunnel: w671 -> [w673]
          stop <- w687 stop-if-true
          # "Stop at LS"
          # "Send command and get position"
          n264 = local read "Travel per Pulse (mm)"() -> (w683:dbl)
          n265 = local read "Cur. Pos X"() -> (w677:dbl)
          n266 = local read "Cur. Pos Y"() -> (w676:dbl)
          n267 = call "Sigma_GetPos.vi"("VISA resource name"=w673, "Travel per Pulse (mm)"=w683, "Init Pos X (mm)"=w677, "Init  Pos Y (mm)"=w676, "error in (no error)"=w680) -> ("Pos X (mm)"=w679:dbl, "Pos Y (mm)"=w678:dbl, "VISA resource name out"=w682:refnum<visa-resource-name>, "State String"=w684:string, "error out"=w681:errorcluster)  [unwired: 6 in]
          n268 = local write "Cur. Pos X"(w679) -> ()
          n269 = local write "Cur. Pos Y"(w678) -> ()
          n270 = Wait Until Next ms Multiple(millisecond multiple=u32 250) -> ()  [unwired: 1 out]
          n271 = case shown="\"K\", Default" w684 {
            tunnel: [w690 w695 w700 w705] -> w675
            tunnel: [w689 w694 w699 w704] -> w674
            tunnel: w682 -> [w690 w692 w697 w702]
            tunnel: w681 -> [w689 w691 w696 w701]
            frame "K", Default {
            }
            frame "L" {
              n272 = call "Sigma_Stop.vi"("Axis (1)"="1", "error in (no error)"=w691, "VISA resource name"=w692) -> ("error out"=w694:errorcluster, "VISA resource name out"=w695:refnum<visa-resource-name>)  [unwired: 7 in]
            }
            frame "M" {
              n273 = call "Sigma_Stop.vi"("Axis (1)"="2", "error in (no error)"=w696, "VISA resource name"=w697) -> ("error out"=w699:errorcluster, "VISA resource name out"=w700:refnum<visa-resource-name>)  [unwired: 7 in]
            }
            frame "W" {
              n274 = call "Sigma_Stop.vi"("Axis (1)"="W", "error in (no error)"=w701, "VISA resource name"=w702) -> ("error out"=w704:errorcluster, "VISA resource name out"=w705:refnum<visa-resource-name>)  [unwired: 7 in]
            }
          }
          n275 = Unbundle By Name(w674) -> ("status"=w688:bool)
          n276 = local read "Scan"() -> (w686:bool)
          n277 = Compound Arithmetic op=OR(w688, w686) -> (w687:bool)
        }
      }
      frame True {
        n278 = local read "Step X"() -> (w708:dbl)
        n279 = local read "Travel per Pulse (mm)"() -> (w707:dbl)
        n280 = local read "Cur. Pos Y"() -> (w718:dbl)
        n281 = call "Sigma_TriggerOut.vi"("Axis(1)"=1, "error in (no error)"=w709, "Trigger distance (mm)"=w708, "Travel per Pulse (mm)"=w707, "VISA resource name"=w712) -> ("error out"=w710:errorcluster, "VISA resource name out"=w711:refnum<visa-resource-name>)  [unwired: 5 in]
        n282 = while {
          shift-right: [w738] -> _
          shift-left: TRUE ("Direction (+)") -> [w751]
          tunnel: w718 -> [w750]
          tunnel: [w746] -> w717
          tunnel: w711 -> [w753]
          tunnel: w710 -> [w752]
          tunnel: [w739] -> w715
          tunnel: [w736] -> w714
          tunnel: w707 -> [w727]
          stop <- w746 stop-if-true
          # "5. Stop scan condition"
          # "3. Run Step Y"
          # "2. wait until run to X-length"
          # "1. Move in X axis\n    Invert direction after moved Step Y"
          # "4. Update Y Possition"
          n283 = flat-sequence {
            tunnel: w753 -> [w759]
            tunnel: w752 -> [w758]
            tunnel: w751 -> [w764]
            tunnel: w750 -> [w762]
            tunnel: [w763] -> w726
            tunnel: [w757] -> w724
            tunnel: [w756] -> w722
            tunnel: [w762] -> w720
            tunnel: w727 -> [w755]
            tunnel: w726 -> [w769]
            tunnel: [w769] -> w725
            tunnel: w724 -> [w768]
            tunnel: [w768] -> w723
            tunnel: w722 -> [w767]
            tunnel: [w767] -> w721
            tunnel: w720 -> [w766]
            tunnel: [w766] -> w719
            tunnel: w725 -> [w772]
            tunnel: w723 -> [w777]
            tunnel: w721 -> [w776]
            tunnel: w719 -> [w773]
            tunnel: [w775] -> w745
            tunnel: [w774] -> w744
            tunnel: [w773] -> w740
            tunnel: [w772] -> w738
            tunnel: [w825] -> w735
            tunnel: w745 -> [w825]
            tunnel: [w824] -> w733
            tunnel: w744 -> [w824]
            tunnel: [w823] -> w731
            tunnel: w740 -> [w823]
            tunnel: w735 -> [w833]
            tunnel: [w833] -> w734
            tunnel: w733 -> [w832]
            tunnel: [w832] -> w732
            tunnel: w731 -> [w827]
            tunnel: [w828] -> w730
            tunnel: [w843] -> w749
            tunnel: [w842] -> w748
            tunnel: w734 -> [w839]
            tunnel: w732 -> [w838]
            tunnel: w730 -> [w835]
            tunnel: w749 -> [w857]
            tunnel: w748 -> [w856]
            tunnel: [w855] -> w741
            tunnel: [w854] -> w737
            tunnel: [w906] -> w743
            tunnel: [w905] -> w742
            tunnel: w741 -> [w905]
            tunnel: w737 -> [w906]
            tunnel: [w904] -> w728
            tunnel: w743 -> [w919]
            tunnel: [w920] -> w736
            tunnel: w742 -> [w920]
            tunnel: [w919] -> w739
            tunnel: [w918] -> w729
            tunnel: w728 -> [w918]
            frame #0 {
              n284 = local read "X-length"() -> (w761:dbl)
              n285 = local write "Move X"(FALSE ("Move X")) -> ()
              n286 = Not(x=w764) -> (.not. x?=w763:bool)
              n287 = call "Sigma_MoveAbs.vi"("Direction (+)"=w763, "Axis (1)"=1, "error in (no error)"=w758, "Travel (1mm)"=w761, "Travel per Pulse (0.004mm)"=w755, "VISA resource name"=w759) -> ("error out"=w756:errorcluster, "VISA resource name out"=w757:refnum<visa-resource-name>)  [unwired: 4 in]
            }
            frame #1 {
              n288 = Wait (ms)(milliseconds to wait=10.0 ("y")) -> ()  [unwired: 1 out]
            }
            frame #2 {
              n289 = local read "Cur. Pos X"() -> (w770:dbl)
              n290 = local read "Cur. Pos Y"() -> (w771:dbl)
              n291 = while {
                tunnel: w777 -> [w790]
                tunnel: w776 -> [w791]
                tunnel: [w789] -> w775
                tunnel: [w788] -> w774
                shift-right: [w782] -> _
                shift-left: w771 -> [w781]
                shift-right: [w783] -> _
                shift-left: w770 -> [w780]
                tunnel: w770 -> [w779]
                stop <- w798 stop-if-true
                # "Stop at LS"
                # "Send command and get position"
                n292 = local read "Travel per Pulse (mm)"() -> (w794:dbl)
                n293 = local read "X-length"() -> (w786:dbl)
                n294 = Wait Until Next ms Multiple(millisecond multiple=u32 100) -> ()  [unwired: 1 out]
                n295 = call "Sigma_GetPos.vi"("VISA resource name"=w790, "Travel per Pulse (mm)"=w794, "Init Pos X (mm)"=w780, "Init  Pos Y (mm)"=w781, "error in (no error)"=w791) -> ("Pos X (mm)"=w783:dbl, "Pos Y (mm)"=w782:dbl, "VISA resource name out"=w793:refnum<visa-resource-name>, "State String"=w795:string, "error out"=w792:errorcluster)  [unwired: 6 in]
                n296 = Subtract(x=w779, y=w783) -> (x-y=w785:dbl)
                n297 = local write "Cur. Pos X"(w783) -> ()
                n298 = local write "Cur. Pos Y"(w782) -> ()
                n299 = Absolute Value(x=w785) -> (abs(x)=w787:dbl)
                n300 = local write "Move X"(TRUE ("Move X")) -> ()
                n301 = Greater Or Equal?(x=w787, y=w786) -> (x >= y?=w784:bool)
                n302 = local read "Stop Scan"() -> (w797:bool)
                n303 = case shown="\"K\", Default" w795 {
                  tunnel: [w801 w806 w811 w816] -> w789
                  tunnel: [w800 w805 w810 w815] -> w788
                  tunnel: w793 -> [w801 w803 w808 w813]
                  tunnel: w792 -> [w800 w802 w807 w812]
                  frame "K", Default {
                  }
                  frame "L" {
                    n304 = call "Sigma_Stop.vi"("Axis (1)"="1", "error in (no error)"=w802, "VISA resource name"=w803) -> ("error out"=w805:errorcluster, "VISA resource name out"=w806:refnum<visa-resource-name>)  [unwired: 7 in]
                  }
                  frame "M" {
                    n305 = call "Sigma_Stop.vi"("Axis (1)"="2", "error in (no error)"=w807, "VISA resource name"=w808) -> ("error out"=w810:errorcluster, "VISA resource name out"=w811:refnum<visa-resource-name>)  [unwired: 7 in]
                  }
                  frame "W" {
                    n306 = call "Sigma_Stop.vi"("Axis (1)"="W", "error in (no error)"=w812, "VISA resource name"=w813) -> ("error out"=w815:errorcluster, "VISA resource name out"=w816:refnum<visa-resource-name>)  [unwired: 7 in]
                  }
                }
                n307 = Unbundle By Name(w788) -> ("status"=w799:bool)
                n308 = Compound Arithmetic op=OR(w799, w797, w784) -> (w798:bool)
              }
            }
            frame #3 {
              n309 = local read "1 Rate"() -> (w821:dbl)
              n310 = local read "Travel per Pulse (mm)"() -> (w822:dbl)
              n311 = local write "Move X"(FALSE ("Move X")) -> ()
              n312 = Divide(x=w821, y=w822) -> (x/y=w818:dbl)
              n313 = Add(x=w818, y=100.0) -> (x+y=w820:dbl)
              n314 = Wait (ms)(milliseconds to wait=w820) -> ()  [unwired: 1 out]
            }
            frame #4 {
              n315 = local read "Y-length"() -> (w826:dbl)
              n316 = local read "Cur. Pos Y"() -> (w831:dbl)
              n317 = Subtract(x=w831, y=w827) -> (x-y=w830:dbl)
              n318 = Absolute Value(x=w830) -> (abs(x)=w829:dbl)
              n319 = Greater Or Equal?(x=w829, y=w826) -> (x >= y?=w828:bool)
            }
            frame #5 {
              # "Stop Y"
              n320 = local read "Step Y"() -> (w841:dbl)
              n321 = local read "Y-length"() -> (w840:dbl)
              n322 = local read "Stop Scan"() -> (w837:bool)
              n323 = Greater Or Equal?(x=w841, y=w840) -> (x >= y?=w836:bool)
              n324 = Compound Arithmetic op=OR(w835, w836, w837) -> (w834:bool)
              n325 = case shown="False" w834 {
                tunnel: [w848 w853] -> w843
                tunnel: [w847 w852] -> w842
                tunnel: w839 -> [w845 w853]
                tunnel: w838 -> [w844 w852]
                frame False {
                  n326 = local read "Travel per Pulse (mm)"() -> (w846:dbl)
                  n327 = local read "Step Y"() -> (w850:dbl)
                  n328 = call "Sigma_MoveAbs.vi"("Axis (1)"=2, "error in (no error)"=w844, "Travel (1mm)"=w850, "Travel per Pulse (0.004mm)"=w846, "VISA resource name"=w845) -> ("error out"=w847:errorcluster, "VISA resource name out"=w848:refnum<visa-resource-name>)  [unwired: 5 in]
                }
                frame True {
                  n329 = local write "Stop Scan"(TRUE ("Stop Scan")) -> ()
                }
              }
            }
            frame #6 {
              n330 = disable-structure shown="Disabled" {
                disable-tunnel: w857 -> [w863 w903]
                disable-tunnel: w856 -> [w862 w902]
                disable-tunnel: [w861 w902] -> w855
                disable-tunnel: [w860 w903] -> w854
                frame Disabled {
                  n331 = local read item#-1() -> (w859)
                  n332 = local read item#-1() -> (w858)
                  n333 = while {
                    tunnel: w863 -> [w875]
                    tunnel: w862 -> [w876]
                    tunnel: [w874] -> w860
                    tunnel: [w873] -> w861
                    shift-right: [w868] -> _
                    shift-left: w858 -> [w865]
                    shift-right: [w867] -> _
                    shift-left: w859 -> [w866]
                    tunnel: w858 -> [w864]
                    stop <- w883 stop-if-true
                    # "Stop at LS"
                    # "Send command and get position"
                    n334 = local read item#-1() -> (w879)
                    n335 = Wait Until Next ms Multiple(millisecond multiple=u32 100) -> ()  [unwired: 1 out]
                    n336 = local read item#-1() -> (w871)
                    n337 = call "Sigma_GetPos.vi"("VISA resource name"=w875, "Travel per Pulse (mm)"=w879, "Init Pos X (mm)"=w866, "Init  Pos Y (mm)"=w865, "error in (no error)"=w876) -> ("Pos X (mm)"=w867:dbl, "Pos Y (mm)"=w868:dbl, "VISA resource name out"=w878:refnum<visa-resource-name>, "State String"=w880:string, "error out"=w877:errorcluster)  [unwired: 6 in]
                    n338 = Subtract(x=w864, y=w868) -> (x-y=w870:dbl)
                    n339 = local write item#-1(w867) -> ()
                    n340 = local write item#-1(w868) -> ()
                    n341 = Absolute Value(x=w870) -> (abs(x)=w872:dbl)
                    n342 = Greater Or Equal?(x=w872, y=w871) -> (x >= y?=w869:bool)
                    n343 = local read "Stop Scan 2"() -> (w882:bool)
                    n344 = case shown="\"K\", Default" w880 {
                      tunnel: [w886 w891 w896 w901] -> w874
                      tunnel: [w885 w890 w895 w900] -> w873
                      tunnel: w878 -> [w886 w888 w893 w898]
                      tunnel: w877 -> [w885 w887 w892 w897]
                      frame "K", Default {
                      }
                      frame "L" {
                        n345 = call "Sigma_Stop.vi"("Axis (1)"="1", "error in (no error)"=w887, "VISA resource name"=w888) -> ("error out"=w890:errorcluster, "VISA resource name out"=w891:refnum<visa-resource-name>)  [unwired: 7 in]
                      }
                      frame "M" {
                        n346 = call "Sigma_Stop.vi"("Axis (1)"="2", "error in (no error)"=w892, "VISA resource name"=w893) -> ("error out"=w895:errorcluster, "VISA resource name out"=w896:refnum<visa-resource-name>)  [unwired: 7 in]
                      }
                      frame "W" {
                        n347 = call "Sigma_Stop.vi"("Axis (1)"="W", "error in (no error)"=w897, "VISA resource name"=w898) -> ("error out"=w900:errorcluster, "VISA resource name out"=w901:refnum<visa-resource-name>)  [unwired: 7 in]
                      }
                    }
                    n348 = Unbundle By Name(w873) -> ("status"=w884:bool)
                    n349 = Compound Arithmetic op=OR(w884, w882, w869) -> (w883:bool)
                  }
                }
                frame Enabled {
                }
              }
            }
            frame #7 {
              n350 = local read "Stop Scan"() -> (w904:bool)
            }
            frame #8 {
              # "waiting for stop speed\naxis 2 + 100ms more"
              n351 = local read "2 Rate"() -> (w910:dbl)
              n352 = local read "Travel per Pulse (mm)"() -> (w909:dbl)
              n353 = local read "Step Y"() -> (w917:dbl)
              n354 = local read "2 Max"() -> (w916:dbl)
              n355 = Compound Arithmetic op=MULTIPLY(w910, invert w909, 2.0 ("value")) -> (w907:dbl)
              n356 = Compound Arithmetic op=MULTIPLY(w917, invert w916, 1000.0 ("value")) -> (w914:dbl)
              n357 = Add(x=w907, y=w914) -> (x+y=w913:dbl)
              n358 = Add(x=w913, y=100.0) -> (x+y=w911:dbl)
              n359 = Wait (ms)(milliseconds to wait=w911) -> ()  [unwired: 1 out]
            }
          }
          n360 = Unbundle By Name(w736) -> ("status"=w747:bool)
          n361 = Compound Arithmetic op=OR(w747, w729) -> (w746:bool)
        }
        "Move X" <- w713
      }
    }
  }
  n362 = call <vilib>:"Simple Error Handler.vi"() -> ()  [unwired: 5 in, 5 out]
